vi "TI sbRIO Main (FPGA).vi"() -> ()   [LabVIEW 2019]
uses:
  <userlib>/_NI SPI IP/FPGA/Controllers/Public/Transfer Settings.ctl
  Type Defs/Diagnostic Mode.ctl
  Controls/SPI Channels.ctl
  <vilib>/Platform/TimedLoop/XDataNode/timing_clust.ctl
  <vilib>/Platform/TimedLoop/XDataNode/nitl_modes.ctl
  <vilib>/Platform/TimedLoop/XDataNode/wakeup.ctl
  <vilib>/rvi/FXPMathLib/FxpDiv/subVIs/nifxpmath_Div_SimConfig.ctl
  <vilib>/rvi/FXPMathLib/basic elements/FxpIntAccumulator/subVIs/nifxpmath_IntAccumulator_SimConfig.ctl
  <vilib>/rvi/FXPMathLib/FxpSqrt/subVIs/nifxpmath_Sqrt_SimConfig.ctl
  <vilib>/fxp/LVFixedPointOverflowPolicyTypeDef.ctl
  <userlib>/_NI SPI IP/FPGA/Controllers/Public/Spi Master Inputs.ctl
  <vilib>/rvi/Emulation/niFpgaGetClockAttributes.vi
  <vilib>/rvi/Emulation/niFpgaSctlEmulationGetInTimedLoop.vi
  <vilib>/rvi/Emulation/niFpgaEmulationReportErrorSimple.vi
  <vilib>/rvi/eio/common/nirviEmuTemplateMethod_errors.vi
  Onboard AIs Global.vi
  <vilib>/rvi/Emulation/niFpgaProcessEmulError.vi
  <vilib>/rvi/Emulation/niFpgaCriticalErrorInLSC.vi
  ADC AI Global.vi
  <vilib>/rvi/FXPMathLib/FxpDiv/simVIs/DllFxpDivTemp_sub.vi
  <vilib>/rvi/DataTransferAndStorage/Container/Common/niFpgaContainerExecOnDevCompGetState.vi
  <vilib>/rvi/Emulation/niFpgaEmulationIsFPGAContextNoSignature.vi
  <vilib>/rvi/errors/niFpgaSetErrorForExecOnDevCompSimple.vi
  <vilib>/rvi/eio/common/nirviEmuReportErrorAndStop.vi
  <vilib>/rvi/DataTransferAndStorage/Container/Common/niFpgaContainerGetUniqueNameForEmu.vi
  <vilib>/rvi/FIFO/Fifo_Resource/nirvififoEmulationSetSize.vi
  <vilib>/rvi/FIFO/Fifo_Resource/nirviFifoEmulationQueueMgr.vi
  <instcachedir>/0/nirviFifoEmulationQueueMgr_E5CAEC123FF24DC58D834DCA3CDAA9B5.lvgen/nirviFifoEmulationQueueMgr_E5CAEC123FF24DC58D834DCA3CDAA9B5_000.vi
  <vilib>/rvi/FIFO/Fifo_Resource/nirvififoEmulationDetermineInputValidOut.vi
  <vilib>/rvi/FIFO/Fifo_Resource/nirvififoEmulationCreateLock.vi
  <vilib>/rvi/FIFO/Fifo_Resource/nirvififoEmulationObtainLock.vi
  <vilib>/rvi/FIFO/Fifo_Resource/nirvififoEmulationReleaseLock.vi
  <vilib>/rvi/occurrence/nirviWaitOnOccurrenceBase.vi
  <vilib>/rvi/errors/nirviReportUnexpectedCaseInternalError.vi
  <vilib>/rvi/errors/nirviReportUnexpectedCaseInternalError (U32).vi
  <vilib>/Utility/error.llb/Clear Errors.vi
  <vilib>/rvi/interface/RandomDataEmulation/niFpgaRandomDataHandleErrors.vi
  Diagnostic Global.vi
  Diagnostic Global (U32).vi
  Flow Frequencies Global.vi
  ADC AI Global (Avg).vi
  <vilib>/rvi/Analysis/common/codeGenErrors/XNode/niFpgaXNodeCodeGenErrorHandle.vi
  <vilib>/rvi/FXPMathLib/basic elements/FxpIntAccumulator/simVIs/DllFxpIntAccumulator_sub.vi
  <vilib>/rvi/FXPMathLib/FxpSqrt/simVIs/DllSqrtTemp_sub.vi
  Pump Currents Global.vi
  ADC AI Global (U32).vi
  <vilib>/eio/EIONode/EIONode.xnode
  <vilib>/rvi/FXPMathLib/FxpDiv/XNode/nifxpmath_Div.xnode
  <vilib>/rvi/DataTransferAndStorage/Container/XNode/niFpgaContainer.xnode
  <vilib>/rvi/FIFO/Fifo_Resource/niFpgaFifoEmulationRefIn.vi
  <vilib>/rvi/FXPMathLib/FxpMul/XNode/nifxpmath_Multiplier.xnode
  <vilib>/rvi/FXPMathLib/FxpAdd/XNode/nifxpmath_Add.xnode
  <vilib>/rvi/Analysis/measure/butterworth/XNode/niFpgaButterworthFilter.xnode
  <vilib>/rvi/Analysis/measure/dc-rms/XNode/niFpgaDC-RMS.xnode
  <vilib>/Platform/TimedLoop/XDataNode/XDataNode.xnode
  <vilib>/rvi/FXPMathLib/basic elements/FxpIntAccumulator/XNode/nifxpmath_IntAccumulator.xnode
  <vilib>/rvi/FXPMathLib/FxpSqrt/XNode/nifxpmath_Sqrt.xnode
  <vilib>/rvi/interface/RandomDataEmulation/nirviRandomDataFpgaReadWriteTemplate.vi
  <vilib>/eio/EIOMethodNode/EIOMethodNode.xnode
  <vilib>/rvi/FXPMathLib/sim/FxpSim.dll
  <vilib>/Platform/TimedLoop/XDataNode/XDNodeRunTimeDep.lvlib
  <userlib>/_NI SPI IP/FPGA/Controllers/NI SPI IP FPGA.lvlib
panel:
  out "Pump Cmds":fxp<+/-,28,17>[](array[numeric])
  in  "Pumps Present":bool[](array[boolean])=[FALSE, FALSE, FALSE, FALSE, FALSE, FALSE]
  in  "Pump Cmds (Duty)":u32[](array[numeric])=[0, 0, 0, 0, 0, 0]
  in  "Debug Restarts":bool
  out "Pump No Starts":u32[](array[numeric])
  in  "Initial No Starts":u32[](array[numeric])=[0, 0, 0, 0, 0, 0]
  in  "Pump Start Time":u32
  out "Restarts":i32[](array[numeric])
  out "Cmd Pump Starts":u32[](array[numeric])
  in  "Stop Command":i32
  in  "Initial Cmd Starts":u32[](array[numeric])=[0, 0, 0, 0, 0, 0]
  in  "Ctrl Currents":fxp<+/-,28,17>[](array[numeric])=[0.0, 0.0, 0.0, 0.0, 0.0, 0.0]
  in  "Initial Acutal Starts":u32[](array[numeric])=[0, 0, 0, 0, 0, 0]
  in  "Power Relays":bool[](array[boolean])=[FALSE, FALSE, FALSE, FALSE, FALSE, FALSE]
  out "Actual Pump Starts":u32[](array[numeric])
  out "Timers (ms)":u32[](array[numeric])
  out "Pump On States":bool[](array[boolean])
  in  "Off Current Thresh":fxp<+/-,28,17>
  in  "Min Off Time":u32
  in  "On Current Thresh":fxp<+/-,28,17>
  in  "Min On Time":u32
  in  "Reset Pump Starts":bool
  in  "Pump Starts Enable":bool
  in  "Diag Max Period (ticks)":u32
  in  "Diagnostic Mode":T1=enum."PSA"
  in  "Duty (Ticks)":i32[](array[numeric])=[0, 0, 0, 0, 0, 0]
  out "Elapsed Times OUT":fxp<+,40,40>[](array[numeric])
  out "Data OUT":fxp<+/-,28,17>[](array[numeric])
  in  "Diagnostic Filter":u16=5
  in  "Invert Diagnostic":bool
  in  "Diagnostic Freq Coeff":i32
  in  "Count Off-Time":bool
  in  "Elapsed Times":fxp<+,40,40>[](array[numeric])=[0.0, 0.0, 0.0, 0.0, 0.0, 0.0]
  in  "ADC Init":bool=TRUE
  in  "FFT_Amp?":bool=TRUE
  in  "Max Period (ticks)":u32
  in  "Freq Flow?":bool
  in  "Divide Value":u8=1
  in  "Current Threshold":fxp<+,26,7>=1.0 format="%#_22g"
  in  "Enable Timers":bool[](array[boolean])=[FALSE, FALSE, FALSE, FALSE, FALSE, FALSE]
  in  "PumpCurrentM":fxp<+/-,16,9>=-60.0 format="%#_25g"
  in  "PumpCurrentB":fxp<+/-,16,9>=-60.0 format="%#_25g"
  in  "InvertPWM?":bool
  in  "DIO25":bool
  in  "DIO24":bool
  out "DIO23":bool
  in  "DIO22":bool
  in  "DIO21":bool
  in  "DIO20":bool
  in  "DIO19":bool
  in  "DIO18":bool
  in  "DIO17":bool
  in  "DIO16":bool
  in  "DIO15":bool
  in  "DIO14":bool
  in  "DIO13":bool
  in  "DIO12":bool
  out "ADC Read Data":u64 format="%.0x"
  in  "ADC CS Mode":enum16{"All", "CS0", "CS1"}(ring)
  in  "ADC Trigger":bool=TRUE
  in  "ADC SPI Settings":T2 {"Direction Change Bit" max=64 step=1; "Transfer Length (bits)" min=1 max=64 step=1}
  in  "ADC Data In":u64 format="%.0x"
  in  "ADC Conversion Request":bool
  in  "ADC Manual":bool
  in  "Brushless":bool
  in  "AI Divisor":u32
  in  "AO3":fxp<+/-,20,5>
  in  "AO2":fxp<+/-,20,5>
  in  "Pressure Cmd":fxp<+/-,20,5>
  in  "PS Cmd":fxp<+/-,20,5>
  in  "Loop Timer (uSec)":u32=100
  in  "Timer Resets":bool[](array[boolean])=[FALSE, FALSE, FALSE, FALSE, FALSE, FALSE]
  in  "PWM Period (Ticks)":u32=40000000
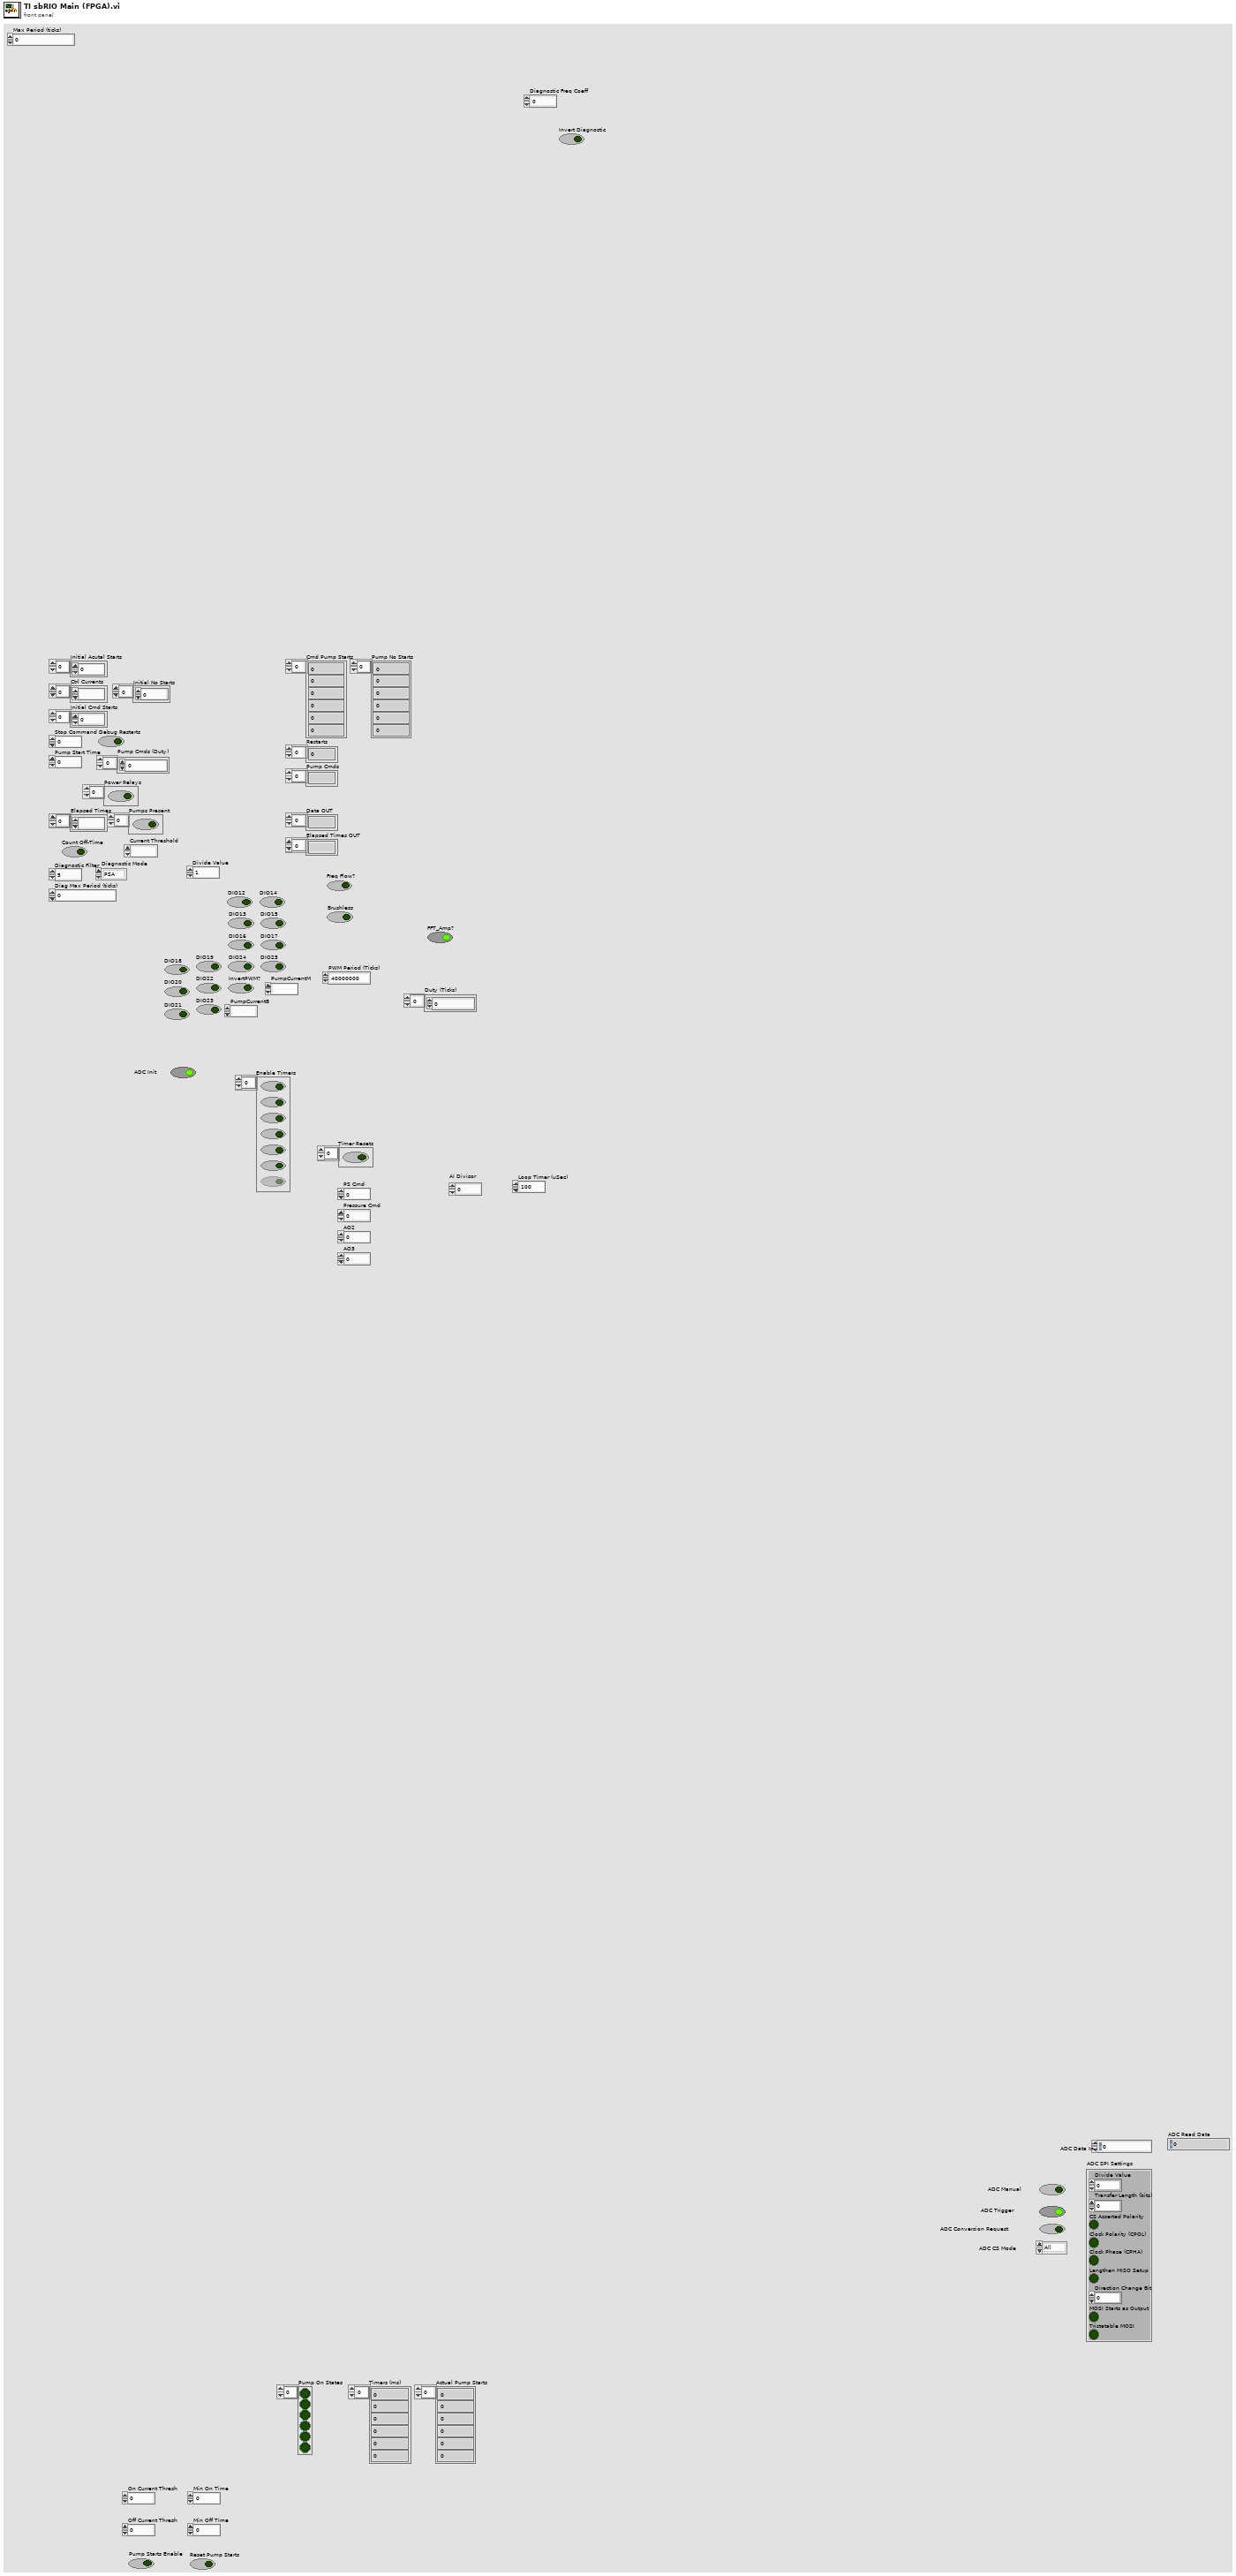
[diagram p1: front panel]
types:
  T1 = typedef "Diagnostic Mode.ctl" = enum16{"None", "PSA", "CMFB"}
  T2 = typedef "NI SPI IP FPGA.lvlib/Transfer Settings.ctl" = cluster{"Divide Value":u8, "Transfer Length (bits)":u8, "CS Asserted Polarity":bool, "Clock Polarity (CPOL)":bool, "Clock Phase (CPHA)":bool, "Lengthen MISO Setup":bool, "Direction Change Bit":u8, "MOSI Starts as Output":bool, "Tristatable MOSI":bool}
  T3 = typedef "SPI Channels.ctl" = cluster{"CS":refnum<k21>, "CLK":refnum<k21>, "MOSI":refnum<k21>, "MISO":refnum<k21>}
  T4 = typedef "XDNodeRunTimeDep.lvlib/timing_clust.ctl" = cluster{"Expected End [f-1]":u64, "Actual End [f-1]":u64, "Finished Late? [f-1]":bool, "Expected End [i-1]":u64, "Actual End [i-1]":u64, "Finished Late? [i-1]":bool, "Expected Start [i]":u64, "Actual Start [i]":u64, "Expected Start [f]":u64, "Actual Start [f]":u64, "Source Name":string, "Structure Name":string, "Period":i64, "Deadline":i64, "Offset":i64, "Start":i64, "Priority":i32, "Timeout":i32, "Mode":T5, "Wakeup Reason":T6, "Error":errorcluster, "Source Type":string, "Secondary Source Type":string, "Global End Time":u64, "Global Start Time":u64, "Frame Duration":u64, "Iteration Duration":u64, "Assigned CPU":i32, "I/O Scan Engine Mode":u32}
  T5 = typedef "XDNodeRunTimeDep.lvlib/nitl_modes.ctl" = enum32{"No Change", "Process missed periods, maintain original phase", "Discard missed periods, maintain original phase", "Process missed periods, ignore original phase", "Discard missed periods, ignore original phase"}
  T6 = typedef "XDNodeRunTimeDep.lvlib/wakeup.ctl" = enum32{"Normal", "Aborted", "Asynchronous wakeup", "Timing source error", "Timed loop error", "Timeout"}
  T7 = typedef "NI SPI IP FPGA.lvlib/Spi Master Inputs.ctl" = cluster{"MISO":bool}
  T8 = typedef "NI SPI IP FPGA.lvlib/Spi Master Outputs.ctl" = cluster{"Chip Select":bool, "Clock":bool, "MOSI":bool, "MOSI OE":bool}
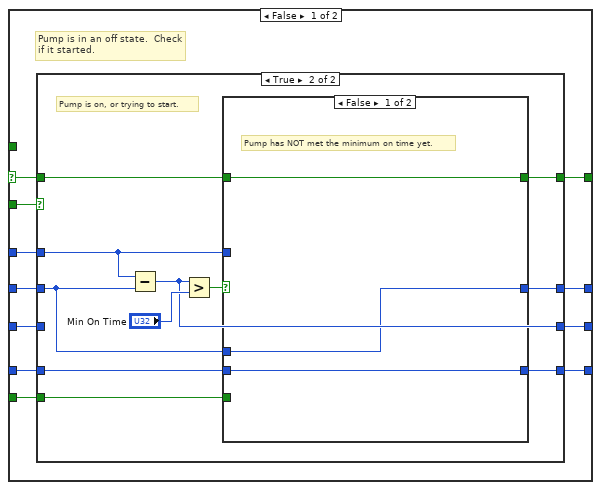
[diagram p6: hidden frame]
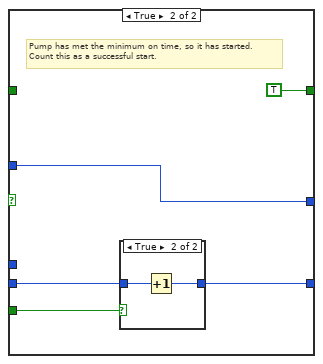
[diagram p8: hidden frame]
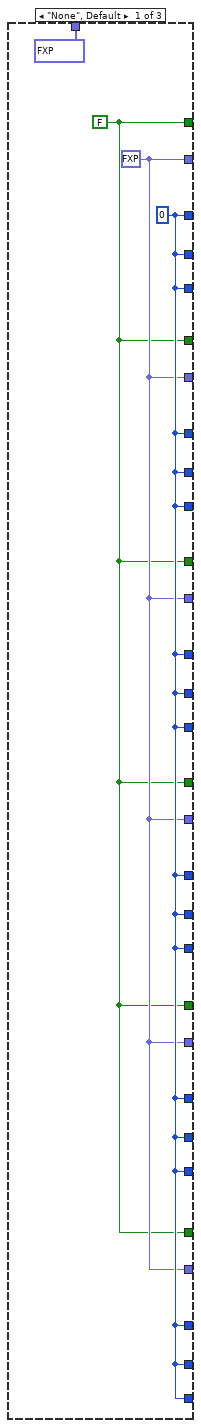
[diagram p12: hidden frame]
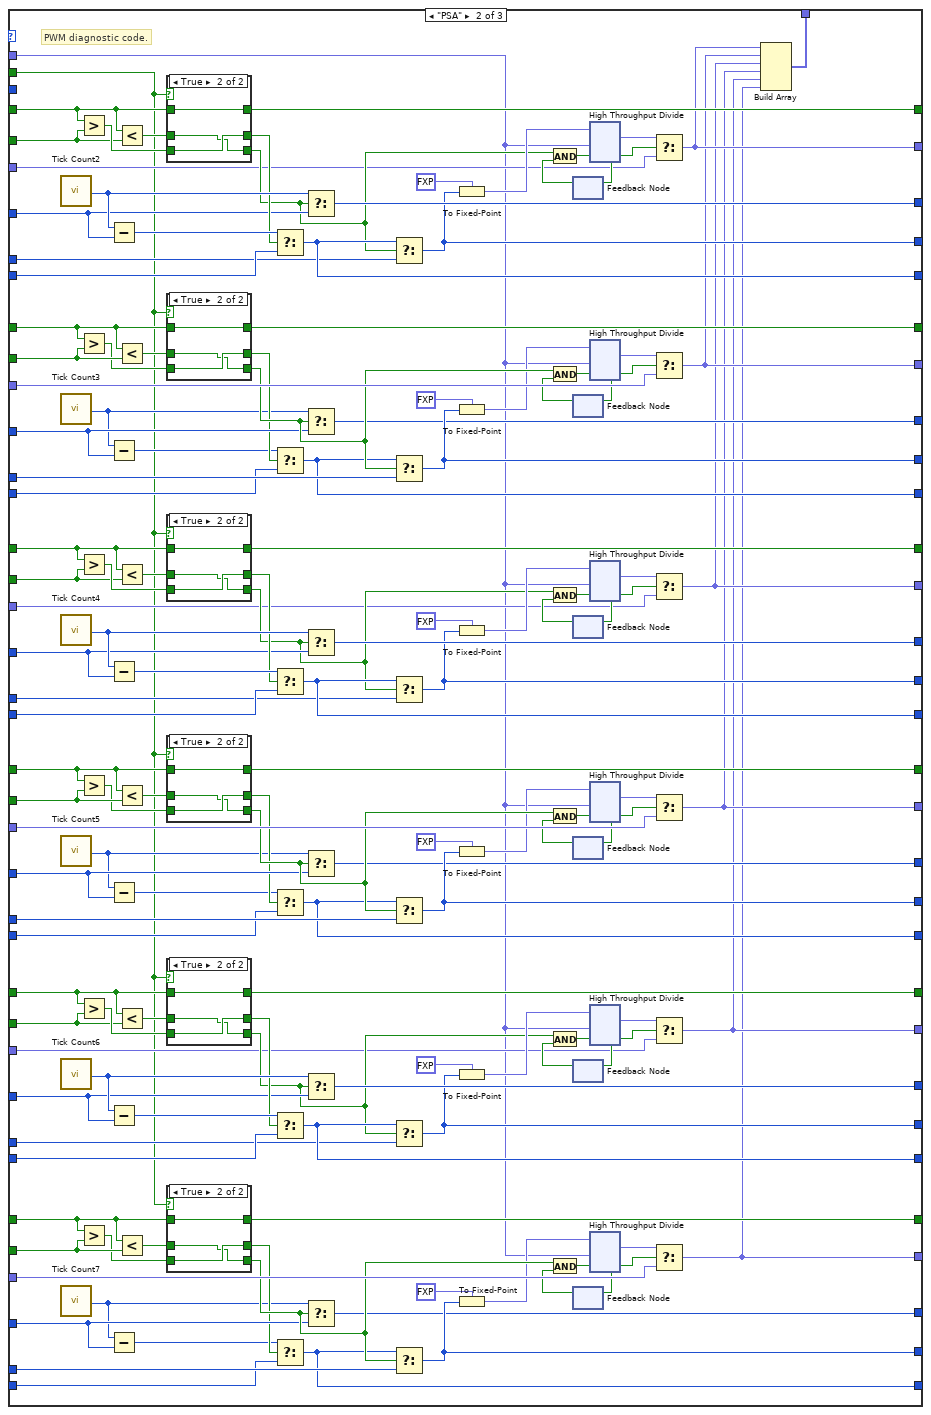
[diagram p13: hidden frame]
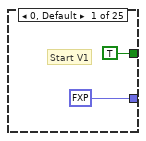
[diagram p20: hidden frame]
diagram:
  w4 = bool[] [FALSE, FALSE, FALSE, FALSE, FALSE, FALSE]  # Pump Triggered
  w10 = bool[] [FALSE, FALSE, FALSE, FALSE, FALSE, FALSE]  # Pump On States
  w41 = refnum<k21> "RMC/DIO60"  # CONVST
  w42 = refnum<k21> "RMC/DIO59"  # CDI
  w43 = refnum<k21> "RMC/DIO58"  # CS1
  w47 = u8 31 ("Sample Divisor")
  # "Pump Start Monitor (for finding restarts)."
  # "DMA for crash files."
  # "Main source of data for RT."
  # "Pump Phase Current and Elapsed Times."
  # "PWM Outputs for Controller Command."
  # "Signal Averaging."
  # "FFT for Pump Speed."
  # "Pump Controller Diagnostics."
  # "Turbine Flow Meters."
  # "Control Signals"
  # "4x ADC\n\nAI16\tPump Current 1\nAI17\tPump Current 2\nAI18\tPump Current 3\nAI19\tPump Current 4\nAI20\tPump Current 5\nAI21\tPump Current 6\nAI22\tController Current 1\nAI23\tController Current 2\nAI24\tController Current 3\nAI25\tController Current 4\nAI26\tController Current 5\nAI27\tController Current 6\nAI28\tTemp 1\nAI29\tTemp 2\nAI30\tPump Pressure 1\nAI31\tPump Pressure 2\nAI32\tPump Pressure 3\nAI33\tPump Pressure 4\nAI34\tPump Pressure 5\nAI35\tPump Pressure 6\nAI36\tPump Flow 1\nAI37\tPump Flow 2\nAI38\tPump Flow 3\nAI39\tPump Flow 4\nAI40\tPump Flow 5\nAI41\tPump Flow 6\nAI42\tSpare\nAI43\tSpare\nAI44\tSpare\nAI45\tSpare\nAI46\tSpare\nAI47\tSpare"
  # "Onboard\n\nAI0/8\tVoltage 1\nAI1/9\tVoltage 2\nAI2/10\tVoltage 3\nAI3/11\tVoltage 4\nAI4/12\tVoltage 5\nAI5/13\tVoltage 6\nAI6\tSpare\nAI14\tSpare\nAI7\tSpare\nAI15\tPower Supply Sense"
  # "This code was created to use\nwith an 8ch analog input to SPI\nchip (ADS8332IPW)."
  # "Explanation for Rounding http://www.eetimes.com/document.asp?doc_id=1274485&page_number=1"
  # "Explanation of Saturation vs. wrapping:   http://www.mathworks.com/help/fixedpoint/ug/saturation-and-wrapping.html\n If scale is 0 to 8 and value is -2               Saturation: 0    Wrapping:  6"
  n1 = node-c288() -> (w32:T4)  [unwired: 1 in]
  n2 = node-c288() -> (w30:T4)  [unwired: 1 in]
  n3 = Unbundle By Name(T3 {"CS"="RMC/DIO57", "CLK"="RMC/DIO54", "MOSI"="RMC/DIO56", "MISO"="RMC/DIO55"} ("SPI Channels")) -> ("CS"=w34:refnum<k21>, "CLK"=w35:refnum<k21>, "MOSI"=w36:refnum<k21>, "MISO"=w37:refnum<k21>)
  n4 = call "Tick Count8"() -> ("Tick Count(mSec)"=w7:u32)
  n5 = timed-loop {
    timing: w32 -> [_]
    timing-out: [_] -> w31
    stop <- FALSE stop-if-true
    n6 = Index Array(array="Power Relays") -> (element #1=w57:bool, element #2=w56:bool, element #3=w55:bool, element #4=w54:bool, element #5=w53:bool, element #6=w52:bool)  [unwired: 6 in]
    n7 = xnode "FPGA I/O Node"("RMC/DIO6"=w57, "RMC/DIO7"=w56, "RMC/DIO8"=w55, "RMC/DIO9"=w54, "RMC/DIO10"=w53, "RMC/DIO11"=w52, "RMC/DIO12"="DIO12", "RMC/DIO13"="DIO13", "RMC/DIO14"="DIO14", "RMC/DIO15"="DIO15", "RMC/DIO16"="DIO16", "RMC/DIO17"="DIO17", "RMC/DIO18"="DIO18", "RMC/DIO19"="DIO19", "RMC/DIO20"="DIO20", "RMC/DIO21"="DIO21", "RMC/DIO22"="DIO22", "RMC/DIO24"="DIO24", "RMC/DIO25"="DIO25") -> ("RMC/DIO23"=→"DIO23":bool)  [unwired: 21 in, 21 out]
  }
  n8 = timed-loop {
    timing: w30 -> [_]
    timing-out: [_] -> w29
    shift-right: [w200] -> _
    shift-left: u32 0 ("f") -> [w199]
    shift-right: [w82] -> _
    shift-left: fxp<+/-,28,17> 0.0 ("AI0") -> [w194]
    shift-right: [w169] -> _
    shift-left: u32 0 ("f") -> [w170]
    shift-right: [w81] -> _
    shift-left: fxp<+/-,28,17> 0.0 ("AI0") -> [w175]
    shift-right: [w160] -> _
    shift-left: u32 0 ("f") -> [w159]
    shift-right: [w80] -> _
    shift-left: fxp<+/-,28,17> 0.0 ("AI0") -> [w154]
    shift-right: [w129] -> _
    shift-left: u32 0 ("f") -> [w130]
    shift-right: [w79] -> _
    shift-left: fxp<+/-,28,17> 0.0 ("AI0") -> [w135]
    shift-right: [w120] -> _
    shift-left: u32 0 ("f") -> [w119]
    shift-right: [w78] -> _
    shift-left: fxp<+/-,28,17> 0.0 ("AI0") -> [w114]
    shift-right: [w89] -> _
    shift-left: u32 0 ("f") -> [w90]
    shift-right: [w77] -> _
    shift-left: fxp<+/-,28,17> 0.0 ("AI0") -> [w95]
    stop <- FALSE stop-if-true
    w84 = fxp<+,32,32> 40000000.0 ("x")
    n9 = xnode "FPGA I/O Node"() -> ("RMC/DIO32"=w204:bool)  [unwired: 1 in, 1 out]
    n10 = xnode "FPGA I/O Node"() -> ("RMC/DIO33"=w165:bool)  [unwired: 1 in, 1 out]
    n11 = xnode "FPGA I/O Node"() -> ("RMC/DIO34"=w164:bool)  [unwired: 1 in, 1 out]
    n12 = xnode "FPGA I/O Node"() -> ("RMC/DIO35"=w125:bool)  [unwired: 1 in, 1 out]
    n13 = xnode "FPGA I/O Node"() -> ("RMC/DIO36"=w124:bool)  [unwired: 1 in, 1 out]
    n14 = xnode "FPGA I/O Node"() -> ("RMC/DIO37"=w85:bool)  [unwired: 1 in, 1 out]
    n15 = feedback-in #1(w204) -> ()
    n16 = feedback #1() -> (w203:bool)  [unwired: 1 in]
    n17 = feedback #2() -> (w166:bool)  [unwired: 1 in]
    n18 = feedback-in #2(w165) -> ()
    n19 = feedback #3() -> (w163:bool)  [unwired: 1 in]
    n20 = feedback-in #3(w164) -> ()
    n21 = feedback #4() -> (w126:bool)  [unwired: 1 in]
    n22 = feedback-in #4(w125) -> ()
    n23 = feedback #5() -> (w123:bool)  [unwired: 1 in]
    n24 = feedback-in #5(w124) -> ()
    n25 = feedback #6() -> (w86:bool)  [unwired: 1 in]
    n26 = feedback-in #6(w85) -> ()
    n27 = Increment(x=w199) -> (x+1=w198:u32)
    n28 = Increment(x=w170) -> (x+1=w171:u32)
    n29 = Increment(x=w159) -> (x+1=w158:u32)
    n30 = Increment(x=w130) -> (x+1=w131:u32)
    n31 = Increment(x=w119) -> (x+1=w118:u32)
    n32 = Increment(x=w90) -> (x+1=w91:u32)
    n33 = Greater?(x=w204, y=w203) -> (0:w185:bool)
    n34 = Greater?(x=w165, y=w166) -> (0:w184:bool)
    n35 = Greater?(x=w164, y=w163) -> (0:w145:bool)
    n36 = Greater?(x=w125, y=w126) -> (0:w144:bool)
    n37 = Greater?(x=w124, y=w123) -> (0:w105:bool)
    n38 = Greater?(x=w85, y=w86) -> (0:w104:bool)
    n39 = Greater?(x=w198, y="Max Period (ticks)") -> (0:w202:bool)
    n40 = Greater?(x=w171, y="Max Period (ticks)") -> (0:w167:bool)
    n41 = Greater?(x=w158, y="Max Period (ticks)") -> (0:w162:bool)
    n42 = Greater?(x=w131, y="Max Period (ticks)") -> (0:w127:bool)
    n43 = Greater?(x=w118, y="Max Period (ticks)") -> (0:w122:bool)
    n44 = Greater?(x=w91, y="Max Period (ticks)") -> (0:w87:bool)
    n45 = To Fixed-Point(number=w198) -> (fixed-point=w197:fxp<+,32,32>)  [unwired: 1 in]
    n46 = To Fixed-Point(number=w171) -> (fixed-point=w172:fxp<+,32,32>)  [unwired: 1 in]
    n47 = To Fixed-Point(number=w158) -> (fixed-point=w157:fxp<+,32,32>)  [unwired: 1 in]
    n48 = To Fixed-Point(number=w131) -> (fixed-point=w132:fxp<+,32,32>)  [unwired: 1 in]
    n49 = To Fixed-Point(number=w118) -> (fixed-point=w117:fxp<+,32,32>)  [unwired: 1 in]
    n50 = To Fixed-Point(number=w91) -> (fixed-point=w92:fxp<+,32,32>)  [unwired: 1 in]
    n51 = feedback #7() -> (w186:bool)  [unwired: 1 in]
    n52 = And(x=w185, y=w186) -> (x .and. y?=w187:bool)
    n53 = feedback #8() -> (w183:bool)  [unwired: 1 in]
    n54 = And(x=w184, y=w183) -> (x .and. y?=w182:bool)
    n55 = feedback #9() -> (w146:bool)  [unwired: 1 in]
    n56 = And(x=w145, y=w146) -> (x .and. y?=w147:bool)
    n57 = feedback #10() -> (w143:bool)  [unwired: 1 in]
    n58 = And(x=w144, y=w143) -> (x .and. y?=w142:bool)
    n59 = feedback #11() -> (w106:bool)  [unwired: 1 in]
    n60 = And(x=w105, y=w106) -> (x .and. y?=w107:bool)
    n61 = feedback #12() -> (w103:bool)  [unwired: 1 in]
    n62 = And(x=w104, y=w103) -> (x .and. y?=w102:bool)
    n63 = xnode "High Throughput Divide"("x"=w84, "y"=w197, "input valid"=w187) -> ("x/y"=w193:fxp<+,28,17>, "output valid"=w189:bool, "ready for input"=w188:bool)  [unwired: 1 in]
    n64 = feedback-in #7(w188) -> ()
    n65 = xnode "High Throughput Divide"("x"=w84, "y"=w172, "input valid"=w182) -> ("x/y"=w176:fxp<+,28,17>, "output valid"=w180:bool, "ready for input"=w181:bool)  [unwired: 1 in]
    n66 = feedback-in #8(w181) -> ()
    n67 = xnode "High Throughput Divide"("x"=w84, "y"=w157, "input valid"=w147) -> ("x/y"=w153:fxp<+,28,17>, "output valid"=w149:bool, "ready for input"=w148:bool)  [unwired: 1 in]
    n68 = feedback-in #9(w148) -> ()
    n69 = xnode "High Throughput Divide"("x"=w84, "y"=w132, "input valid"=w142) -> ("x/y"=w136:fxp<+,28,17>, "output valid"=w140:bool, "ready for input"=w141:bool)  [unwired: 1 in]
    n70 = feedback-in #10(w141) -> ()
    n71 = xnode "High Throughput Divide"("x"=w84, "y"=w117, "input valid"=w107) -> ("x/y"=w113:fxp<+,28,17>, "output valid"=w109:bool, "ready for input"=w108:bool)  [unwired: 1 in]
    n72 = feedback-in #11(w108) -> ()
    n73 = xnode "High Throughput Divide"("x"=w84, "y"=w92, "input valid"=w102) -> ("x/y"=w96:fxp<+,28,17>, "output valid"=w100:bool, "ready for input"=w101:bool)  [unwired: 1 in]
    n74 = feedback-in #12(w101) -> ()
    n75 = Select(t=u32 0 ("f"), s=w189, f=w198) -> (s? t:f=w200:u32)
    n76 = Select(t=u32 0 ("f"), s=w180, f=w171) -> (s? t:f=w169:u32)
    n77 = Select(t=u32 0 ("f"), s=w149, f=w158) -> (s? t:f=w160:u32)
    n78 = Select(t=u32 0 ("f"), s=w140, f=w131) -> (s? t:f=w129:u32)
    n79 = Select(t=u32 0 ("f"), s=w109, f=w118) -> (s? t:f=w120:u32)
    n80 = Select(t=u32 0 ("f"), s=w100, f=w91) -> (s? t:f=w89:u32)
    n81 = To Fixed-Point(fixed-point type=fxp<+/-,28,17> 0.0 ("AI0"), number=w193) -> (fixed-point=w191:fxp<+/-,28,17>)
    n82 = To Fixed-Point(fixed-point type=fxp<+/-,28,17> 0.0 ("AI0"), number=w176) -> (fixed-point=w178:fxp<+/-,28,17>)
    n83 = To Fixed-Point(fixed-point type=fxp<+/-,28,17> 0.0 ("AI0"), number=w153) -> (fixed-point=w151:fxp<+/-,28,17>)
    n84 = To Fixed-Point(fixed-point type=fxp<+/-,28,17> 0.0 ("AI0"), number=w136) -> (fixed-point=w138:fxp<+/-,28,17>)
    n85 = To Fixed-Point(fixed-point type=fxp<+/-,28,17> 0.0 ("AI0"), number=w113) -> (fixed-point=w111:fxp<+/-,28,17>)
    n86 = To Fixed-Point(fixed-point type=fxp<+/-,28,17> 0.0 ("AI0"), number=w96) -> (fixed-point=w98:fxp<+/-,28,17>)
    n87 = Or(x=w202, y=w189) -> (x .or. y?=w195:bool)
    n88 = Or(x=w167, y=w180) -> (x .or. y?=w174:bool)
    n89 = Or(x=w162, y=w149) -> (x .or. y?=w155:bool)
    n90 = Or(x=w127, y=w140) -> (x .or. y?=w134:bool)
    n91 = Or(x=w122, y=w109) -> (x .or. y?=w115:bool)
    n92 = Or(x=w87, y=w100) -> (x .or. y?=w94:bool)
    n93 = Select(t=fxp<+/-,28,17> 0.0 ("AI0"), s=w202, f=w191) -> (s? t:f=w196:fxp<+/-,28,17>)
    n94 = Select(t=fxp<+/-,28,17> 0.0 ("AI0"), s=w167, f=w178) -> (s? t:f=w173:fxp<+/-,28,17>)
    n95 = Select(t=fxp<+/-,28,17> 0.0 ("AI0"), s=w162, f=w151) -> (s? t:f=w156:fxp<+/-,28,17>)
    n96 = Select(t=fxp<+/-,28,17> 0.0 ("AI0"), s=w127, f=w138) -> (s? t:f=w133:fxp<+/-,28,17>)
    n97 = Select(t=fxp<+/-,28,17> 0.0 ("AI0"), s=w122, f=w111) -> (s? t:f=w116:fxp<+/-,28,17>)
    n98 = Select(t=fxp<+/-,28,17> 0.0 ("AI0"), s=w87, f=w98) -> (s? t:f=w93:fxp<+/-,28,17>)
    n99 = Select(t=w196, s=w195, f=w194) -> (s? t:f=w82:fxp<+/-,28,17>)
    n100 = Select(t=w173, s=w174, f=w175) -> (s? t:f=w81:fxp<+/-,28,17>)
    n101 = Select(t=w156, s=w155, f=w154) -> (s? t:f=w80:fxp<+/-,28,17>)
    n102 = Select(t=w133, s=w134, f=w135) -> (s? t:f=w79:fxp<+/-,28,17>)
    n103 = Select(t=w116, s=w115, f=w114) -> (s? t:f=w78:fxp<+/-,28,17>)
    n104 = Select(t=w93, s=w94, f=w95) -> (s? t:f=w77:fxp<+/-,28,17>)
    n105 = Build Array(w82, w81, w80, w79, w78, w77) -> (w76:fxp<+/-,28,17>[])
    n106 = global write "Flow Frequencies Global.vi" "Flow Frequencies"(w76) -> ()
  }
  n107 = local read "Duty (Ticks)"() -> (w5:i32[])
  n108 = while {
    shift-right: [w383] -> _
    shift-left: "Elapsed Times" -> [w394]
    shift-right: [w384] -> _
    shift-left: u32[] [0, 0, 0, 0, 0, 0] -> [w385]
    stop <- FALSE stop-if-true
    # "Pump Current\nAI16-21"
    # "from:S 64 44\nto: U 40 40"
    n109 = global read "ADC AI Global.vi" "AI16-47"() -> (w387:fxp<+/-,28,17>[])
    n110 = feedback #13() -> (w392:bool[])  [unwired: 1 in]
    n111 = feedback-in #13("Timer Resets") -> ()
    n112 = Array Subset(array=w387, index=0, length=6) -> (w389:fxp<+/-,28,17>[])
    n113 = Greater?(x="Timer Resets", y=w392) -> (0:w395:bool[])
    n114 = for {
      tunnel: w389 -> [w429] mode=indexing
      tunnel: w395 -> [w431] mode=indexing
      tunnel: [w401] -> w386 mode=indexing
      tunnel: w394 -> [w426] mode=indexing
      tunnel: [w425] -> w383 mode=indexing
      tunnel: "Enable Timers" -> [w420] mode=indexing
      tunnel: w385 -> [w408] mode=indexing
      tunnel: [w403] -> w384 mode=indexing
      tunnel: "Count Off-Time" -> [w399]
      i -> [w430]
      w424 = fxp<+/-,26,7> 0.0 ("out")
      # "Formerly looking for DC signal based on period detection\nNow looking for staying in the 0A range"
      # "Calibration issue should only\nbe if reading is negative at 0A"
      # "30ms calculated as longest waveform period"
      # "RMS vi only outputs positive values, so put back to negative if that's the way it went in.  This fixes a calibration issue."
      # "D2A factor"
      # "Rough scale and offset for\nspeed and RMS measurements."
      n115 = xnode "High Throughput Divide"("x"=w429, "y"=fxp<+,14,14> 13107.0 ("Current Scale")) -> ("x/y"=w423:fxp<+/-,28,17>)
      n116 = xnode ("High Throughput Multiply")("x"=w423, "y"="PumpCurrentM") -> ("x*y"=w422:fxp<+/-,29,10>)
      n117 = xnode ("High Throughput Add")("x"=w422, "y"="PumpCurrentB") -> ("x+y"=w411:fxp<+/-,30,11>)
      n118 = Less?(x=w411, y=fxp<+/-,30,11> 0.25) -> (x < y?=w409:bool)
      n119 = xnode "Butterworth Filter"("input data"=w411) -> ("output data"=w413:fxp<+/-,20,15>)  [unwired: 2 in, 1 out]
      n120 = case shown="True" w409 {
        tunnel: w408 -> [_ w434]
        tunnel: [u32 0 w433] -> w403
        frame False {
        }
        frame True {
          n121 = Increment(x=w434) -> (x+1=w433:u32)
        }
      }
      n122 = To Fixed-Point(fixed-point type=w424, number=w411) -> (fixed-point=w416:fxp<+/-,26,7>)
      n123 = To Fixed-Point(fixed-point type=w424, number=w413) -> (fixed-point=w414:fxp<+/-,26,7>)
      n124 = case shown="False" "Brushless" {
        tunnel: [w435 w436] -> w415
        tunnel: w416 -> [_ w436]
        tunnel: w414 -> [w435 _]
        frame False {
        }
        frame True {
        }
      }
      n125 = Greater?(x=w403, y=u32 300) -> (0:w404:bool)
      n126 = Less Than 0?(x=w415) -> (x < 0?=w407:bool)
      n127 = case shown="0, Default" w430 {
        tunnel: [w490 w600 w710 w820 w930 w1040] -> w417
        tunnel: w415 -> [w489 w599 w709 w819 w929 w1039]
        frame 0, Default {
          n128 = xnode ("DC and RMS Measurements 5")("input data"=w489) -> ("RMS"=w490:fxp<+,26,7>)  [unwired: 1 in, 1 out]
        }
        frame 1 {
          n129 = xnode ("DC and RMS Measurements")("input data"=w599) -> ("RMS"=w600:fxp<+,26,7>)  [unwired: 1 in, 1 out]
        }
        frame 2 {
          n130 = xnode ("DC and RMS Measurements 2")("input data"=w709) -> ("RMS"=w710:fxp<+,26,7>)  [unwired: 1 in, 1 out]
        }
        frame 3 {
          n131 = xnode ("DC and RMS Measurements 3")("input data"=w819) -> ("RMS"=w820:fxp<+,26,7>)  [unwired: 1 in, 1 out]
        }
        frame 4 {
          n132 = xnode ("DC and RMS Measurements 4")("input data"=w929) -> ("RMS"=w930:fxp<+,26,7>)  [unwired: 1 in, 1 out]
        }
        frame 5 {
          n133 = xnode ("DC and RMS Measurements 6")("input data"=w1039) -> ("RMS"=w1040:fxp<+,26,7>)  [unwired: 1 in, 1 out]
        }
      }
      n134 = And(x=w407, y=w404) -> (x .and. y?=w406:bool)
      n135 = To Fixed-Point(fixed-point type=fxp<+/-,28,17> 0.0 ("out"), number=w417) -> (fixed-point=w418:fxp<+/-,28,17>)
      n136 = case shown="True" w406 {
        tunnel: w418 -> [w437 w439]
        tunnel: [w437 w438] -> w401
        frame False {
        }
        frame True {
          n137 = Negate(x=w439) -> (-x=w438:fxp<+/-,29,18>)
        }
      }
      n138 = Greater?(x=w401, y="Current Threshold") -> (0:w400:bool)
      n139 = Or(x=w400, y=w399) -> (x .or. y?=w398:bool)
      n140 = case shown="True" w431 {
        tunnel: w398 -> [w470 _]
        tunnel: w426 -> [w469 _]
        tunnel: [w468 fxp<+,40,40> 0.0 ("AI0")] -> w425
        tunnel: w420 -> [w467 _]
        frame False {
          n141 = case shown="True" w467 {
            tunnel: w470 -> [_ w474]
            tunnel: w469 -> [w471 w473]
            tunnel: [w471 w472] -> w468
            frame False {
            }
            frame True {
              n142 = case shown="True" w474 {
                tunnel: [w475 w476] -> w472
                tunnel: w473 -> [w475 w478]
                frame False {
                }
                frame True {
                  # "Was: Sat/Trunc       Now:  Wrap/Trunc"
                  # "Greater than 1 amp, so pump is \"on\"."
                  n143 = xnode ("High Throughput Add")("x"=w478, "y"=fxp<+,1,1> 1.0) -> ("x+y"=w476:fxp<+,40,40>)
                }
              }
            }
          }
        }
        frame True {
        }
      }
    }
    n144 = call "Loop Timer"("Count(uSec)"="Loop Timer (uSec)") -> ()  [unwired: 1 out]
    n145 = global write "Pump Currents Global.vi" "Pump Currents"(w386) -> ()
    n146 = local write "Elapsed Times"(w383) -> ()
  }
  n147 = while {
    stop <- FALSE stop-if-true
    n148 = Index Array(array="Duty (Ticks)") -> (element #1=w1154:i32, element #2=w1153:i32, element #3=w1152:i32, element #4=w1151:i32, element #5=w1150:i32, element #6=w1149:i32)  [unwired: 6 in]
    n149 = call "Pulse Width Modulation (FPGA).vi"("PWM Period (Ticks)"="PWM Period (Ticks)", "PWM Duty Cycle (Ticks)"=w1154) -> ("PWM DO"=w1168:bool)  [unwired: 14 in, 3 out]
    n150 = call "Pulse Width Modulation (FPGA).vi"("PWM Period (Ticks)"="PWM Period (Ticks)", "PWM Duty Cycle (Ticks)"=w1153) -> ("PWM DO"=w1167:bool)  [unwired: 14 in, 3 out]
    n151 = call "Pulse Width Modulation (FPGA).vi"("PWM Period (Ticks)"="PWM Period (Ticks)", "PWM Duty Cycle (Ticks)"=w1152) -> ("PWM DO"=w1166:bool)  [unwired: 14 in, 3 out]
    n152 = call "Pulse Width Modulation (FPGA).vi"("PWM Period (Ticks)"="PWM Period (Ticks)", "PWM Duty Cycle (Ticks)"=w1151) -> ("PWM DO"=w1165:bool)  [unwired: 14 in, 3 out]
    n153 = call "Pulse Width Modulation (FPGA).vi"("PWM Period (Ticks)"="PWM Period (Ticks)", "PWM Duty Cycle (Ticks)"=w1150) -> ("PWM DO"=w1164:bool)  [unwired: 14 in, 3 out]
    n154 = call "Pulse Width Modulation (FPGA).vi"("PWM Period (Ticks)"="PWM Period (Ticks)", "PWM Duty Cycle (Ticks)"=w1149) -> ("PWM DO"=w1163:bool)  [unwired: 14 in, 3 out]
    n155 = Exclusive Or(1:"InvertPWM?", 2:w1168) -> (0:w1161:bool)
    n156 = Exclusive Or(1:"InvertPWM?", 2:w1167) -> (0:w1160:bool)
    n157 = Exclusive Or(1:"InvertPWM?", 2:w1166) -> (0:w1159:bool)
    n158 = Exclusive Or(1:"InvertPWM?", 2:w1165) -> (0:w1158:bool)
    n159 = Exclusive Or(1:"InvertPWM?", 2:w1164) -> (0:w1157:bool)
    n160 = Exclusive Or(1:"InvertPWM?", 2:w1163) -> (0:w1156:bool)
    n161 = xnode "FPGA I/O Node"("RMC/DIO0"=w1161, "RMC/DIO1"=w1160, "RMC/DIO2"=w1159, "RMC/DIO3"=w1158, "RMC/DIO4"=w1157, "RMC/DIO5"=w1156) -> ()  [unwired: 7 in, 7 out]
  }
  n162 = node-c288() -> (w45:T4)  [unwired: 1 in]
  n163 = node-c288() -> (w51:T4)  [unwired: 1 in]
  n164 = node-c288() -> (w12:T4)  [unwired: 1 in]
  n165 = Initialize Array(w7, 6 ("dimension size")) -> (w3:u32[])
  n166 = Decrement(x=w47) -> (x-1=w48:u8)
  n167 = timed-loop "4x ADC SPI Loop" {
    shift-right: [w1195] -> _
    shift-left: fxp<+/-,28,17>[] [0.0, 0.0, 0.0, 0.0, 0.0, 0.0, 0.0, 0.0, 0.0, 0.0, 0.0, 0.0, 0.0, 0.0, 0.0, 0.0, 0.0, 0.0, 0.0, 0.0, 0.0, 0.0, 0.0, 0.0, 0.0, 0.0, 0.0, 0.0, 0.0, 0.0, 0.0, 0.0] -> [w1196]
    tunnel: w34 -> [w1194]
    tunnel: w35 -> [w1193]
    tunnel: w36 -> [w1192]
    tunnel: w37 -> [w1191]
    tunnel: w43 -> [w1190]
    tunnel: w41 -> [w1189]
    tunnel: w42 -> [w1188]
    timing: w45 -> [_]
    timing-out: [_] -> w44
    shift-right: [w1177] -> _
    shift-left: u8 2 ("lo(x)") -> [w1178]
    shift-right: [w1174] -> _
    shift-left: u8 0 ("lo(x)") -> [w1175]
    shift-right: [w1171] -> _
    shift-left: u32[] [0, 0, 0, 0, 0, 0, 0, 0, 0, 0, 0, 0, 0, 0, 0, 0, 0, 0, 0, 0, 0, 0, 0, 0, 0, 0, 0, 0, 0, 0, 0, 0] -> [w1172]
    stop <- FALSE stop-if-true
    n168 = flat-sequence {
      tunnel: [w1209] -> w1187
      tunnel: w1196 -> [w1209]
      tunnel: w1194 -> [w1208]
      tunnel: w1193 -> [w1207]
      tunnel: w1192 -> [w1206]
      tunnel: w1191 -> [w1205]
      tunnel: [w1208] -> w1186
      tunnel: [w1207] -> w1185
      tunnel: [w1206] -> w1184
      tunnel: [w1205] -> w1183
      tunnel: w1190 -> [w1204]
      tunnel: w1189 -> [w1203]
      tunnel: w1188 -> [w1202]
      tunnel: [w1204] -> w1182
      tunnel: [w1202] -> w1181
      tunnel: [w1203] -> w1180
      tunnel: [w1201] -> w1179
      tunnel: w1178 -> [w1201]
      tunnel: [w1200] -> w1176
      tunnel: w1175 -> [w1200]
      tunnel: [w1198] -> w1173
      tunnel: w1172 -> [w1198]
      tunnel: w1187 -> [w1254]
      tunnel: [w1253] -> w1195
      tunnel: w1186 -> [w1249]
      tunnel: w1185 -> [w1252]
      tunnel: w1184 -> [w1251]
      tunnel: w1183 -> [w1250]
      tunnel: w1182 -> [w1248]
      tunnel: w1181 -> [_]
      tunnel: w1180 -> [w1234]
      tunnel: w1179 -> [w1235]
      tunnel: [w1229] -> w1177
      tunnel: w1176 -> [w1228]
      tunnel: [w1227] -> w1174
      tunnel: w1173 -> [w1226]
      tunnel: [w1225] -> w1171
      frame #0 {
        # "Message Type Index"
        n169 = case shown="True" "ADC Init" {
          tunnel: w1208 -> [_ w1224]
          tunnel: w1207 -> [_ w1223]
          tunnel: w1206 -> [_ w1222]
          tunnel: w1205 -> [_ w1221]
          tunnel: w1204 -> [_ w1220]
          tunnel: w1203 -> [_ w1219]
          tunnel: w1202 -> [_ w1218]
          frame False {
          }
          frame True {
            w1211 = TRUE ("I/O Item")
            w1216 = TRUE ("Enable")
            n170 = xnode "FPGA I/O Method Node"("FPGA I/O In"=w1219, "Enable"=w1216) -> ("FPGA I/O Out"=w1212:refnum<k21>)
            n171 = xnode "FPGA I/O Method Node"("FPGA I/O In"=w1218, "Enable"=FALSE) -> ()  [unwired: 1 out]
            n172 = xnode "FPGA I/O Method Node"("FPGA I/O In"=w1220, "Enable"=w1216) -> ("FPGA I/O Out"=w1215:refnum<k21>)
            n173 = xnode "FPGA I/O Method Node"("FPGA I/O In"=w1224, "Enable"=w1216) -> ("FPGA I/O Out"=w1214:refnum<k21>)
            n174 = xnode "FPGA I/O Method Node"("FPGA I/O In"=w1223, "Enable"=w1216) -> ()  [unwired: 1 out]
            n175 = xnode "FPGA I/O Method Node"("FPGA I/O In"=w1222, "Enable"=w1216) -> ()  [unwired: 1 out]
            n176 = xnode "FPGA I/O Method Node"("FPGA I/O In"=w1221, "Enable"=FALSE) -> ()  [unwired: 1 out]
            n177 = xnode "FPGA I/O Node"("I/O Item"=w1211, "FPGA I/O In"=w1212, "I/O Item"=w1211, "FPGA I/O In"=w1215, "I/O Item"=w1211, "FPGA I/O In"=w1214) -> ()  [unwired: 3 out]
            n178 = local write "ADC Init"(FALSE ("ADC Init")) -> ()
          }
        }
      }
      frame #1 {
        # "Message Index"
        # "Channel Index"
        # "16 Bits-Send Channel Selection, CS Normal \n42 Bits Assert Conversion Request, CS Not Enabled\n64 Bits - Unassert Conversion, CS Normal"
        # "CONVERSION REQ"
        n179 = xnode "FPGA I/O Node"("FPGA I/O In"=w1250) -> ("I/O Item"=w1255:bool)  [unwired: 1 out]
        n180 = Bundle By Name(cluster=T7 {"MISO"=FALSE} ("spi input"), "MISO"=w1255) -> (w1256:T7)
        n181 = feedback #14(TRUE ("Chip Select")) -> (w1231:bool)
        n182 = case shown="False" "ADC Manual" {
          tunnel: w1231 -> [w1263 w1316]
          tunnel: [w1263 w1315] -> w1237
          tunnel: [w1268 "ADC SPI Settings"] -> w1236
          tunnel: w1235 -> [w1262 _]
          tunnel: [w1264 "ADC Data In"] -> w1232
          tunnel: [w1261 w1311] -> w1229
          tunnel: [w1267 "ADC Conversion Request"] -> w1233
          tunnel: w1228 -> [w1266 _]
          tunnel: [w1265 w1311] -> w1227
          frame False {
            # "Auto Mode"
            n183 = Boolean To (0,1)(Boolean=w1263) -> (0, 1=w1275:i16)
            n184 = To Unsigned Byte Integer(number=w1275) -> (unsigned 8bit integer=w1274:u8)
            n185 = Add(x=w1274, y=w1262) -> (x+y=w1270:u8)
            n186 = Greater?(x=w1270, y=u8 2) -> (0:w1272:bool)
            n187 = Select(t=u8 0 ("y"), s=w1272, f=w1270) -> (s? t:f=w1269:u8)
            n188 = case shown="1" w1269 {
              selector: w1269 -> [w1282 w1288 w1298]
              tunnel: [w1276 w1285 w1292] -> w1268
              tunnel: [TRUE ("I/O Item") FALSE ("I/O Item") TRUE ("I/O Item")] -> w1267
              tunnel: w1266 -> [w1281 w1289 w1297]
              tunnel: [w1281 w1289 w1296] -> w1265
              tunnel: [w1279 u64 0 u64 53248] -> w1264
              tunnel: w1263 -> [_ _ w1300]
              tunnel: w1262 -> [_ _ w1295]
              tunnel: [w1282 w1288 w1299] -> w1261
              tunnel: "Divide Value" -> [w1277 w1287 w1294]
              frame 0, Default {
                # "16 Bits"
                # "Channel Select"
                # "0x#000"
                n189 = Bundle By Name(cluster=T2 {"Divide Value"=1, "Transfer Length (bits)"=16, "CS Asserted Polarity"=FALSE, "Clock Polarity (CPOL)"=TRUE, "Clock Phase (CPHA)"=FALSE, "Lengthen MISO Setup"=FALSE, "Direction Change Bit"=0, "MOSI Starts as Output"=FALSE, "Tristatable MOSI"=FALSE} ("Master Settings 2"), "Divide Value"=w1277) -> (w1276:T2)
                n190 = To Unsigned Quad Integer(1:w1281) -> (0:w1280:u64)
                n191 = Logical Shift(y=i16 12, x=w1280) -> (x << y=w1279:u64)
              }
              frame 1 {
                # "Conversion Request Asserted"
                # "42 Bits"
                # "Dont Care"
                n192 = Bundle By Name(cluster=T2 {"Divide Value"=1, "Transfer Length (bits)"=42, "CS Asserted Polarity"=FALSE, "Clock Polarity (CPOL)"=TRUE, "Clock Phase (CPHA)"=FALSE, "Lengthen MISO Setup"=FALSE, "Direction Change Bit"=0, "MOSI Starts as Output"=FALSE, "Tristatable MOSI"=FALSE} ("Master Settings 2"), "Divide Value"=w1287) -> (w1285:T2)
              }
              frame 2 {
                # "64 Bits"
                # "Read CMD"
                n193 = Bundle By Name(cluster=T2 {"Divide Value"=1, "Transfer Length (bits)"=64, "CS Asserted Polarity"=FALSE, "Clock Polarity (CPOL)"=TRUE, "Clock Phase (CPHA)"=FALSE, "Lengthen MISO Setup"=FALSE, "Direction Change Bit"=0, "MOSI Starts as Output"=FALSE, "Tristatable MOSI"=FALSE} ("Master Settings 2"), "Divide Value"=w1294) -> (w1292:T2)
                n194 = case shown="False" w1300 {
                  tunnel: [w1303 w1307] -> w1299
                  tunnel: w1298 -> [_ w1307]
                  tunnel: w1297 -> [w1304 w1308]
                  tunnel: [w1304 w1305] -> w1296
                  tunnel: w1295 -> [w1303 _]
                  frame False {
                  }
                  frame True {
                    n195 = Increment(x=w1308) -> (x+1=w1306:u8)
                    n196 = case shown="8" w1306 {
                      selector: w1306 -> [w1309 _]
                      tunnel: [w1309 u8 0] -> w1305
                      frame Default {
                      }
                      frame 8 {
                      }
                    }
                  }
                }
              }
            }
          }
          frame True {
            w1311 = u8 0 ("y")
            # "Manual Mode"
            n197 = feedback #15(FALSE) -> (w1320:bool)
            n198 = feedback-in #15("ADC Trigger") -> ()
            n199 = Greater?(x="ADC Trigger", y=w1320) -> (0:w1317:bool)
            n200 = And(x=w1317, y=w1316) -> (x .and. y?=w1315:bool)
          }
        }
        n201 = call <userlib>:"Spi Master.vi"("spi input"=w1256, "start strobe"=w1237, "data to write"=w1232, "MOSI output enable done"=TRUE, "spi transfer settings"=w1236) -> ("spi output"=w1259:T8, "read data valid"=w1230:bool, "read data"=w1244:u64, "ready for input"=w1246:bool)  [unwired: 7 in]
        "ADC Read Data" <- w1244
        n202 = feedback-in #14(w1246) -> ()
        n203 = Unbundle By Name(w1259) -> ("Chip Select"=w1241:bool, "Clock"=w1245:bool, "MOSI"=w1258:bool)
        n204 = case shown="\"All\", Default" "ADC CS Mode" {
          tunnel: w1241 -> [w1322 w1324 w1328]
          tunnel: [TRUE ("Chip Select") w1324 w1327] -> w1240
          tunnel: [w1322 TRUE ("Chip Select") w1326] -> w1239
          tunnel: w1229 -> [_ _ w1330]
          frame "CS1" {
          }
          frame "CS0" {
          }
          frame "All", Default {
            n205 = Equal?(x=w1330, y=u8 1) -> (x = y?=w1325:bool)
            n206 = case shown="False" w1325 {
              tunnel: w1328 -> [w1331 _]
              tunnel: [w1331 w1332] -> w1327
              tunnel: [w1331 w1332] -> w1326
              frame False {
              }
              frame True {
                w1332 = TRUE ("Chip Select")
              }
            }
          }
        }
        n207 = case shown="True" w1230 {
          tunnel: w1244 -> [_ w1341]
          tunnel: w1254 -> [w1334 w1340]
          tunnel: [w1334 w1339] -> w1253
          tunnel: w1232 -> [_ w1338]
          tunnel: w1227 -> [_ w1337]
          tunnel: w1226 -> [w1333 w1336]
          tunnel: [w1333 w1335] -> w1225
          frame False {
          }
          frame True {
            n208 = case shown="53248" w1338 {
              tunnel: w1341 -> [_ w1372]
              tunnel: w1340 -> [w1343 w1371]
              tunnel: [w1343 w1358] -> w1339
              tunnel: w1337 -> [_ w1364]
              tunnel: w1336 -> [w1342 w1357]
              tunnel: [w1342 w1348] -> w1335
              frame Default {
              }
              frame 53248 {
                w1363 = fxp<+/-,28,17> 0.0 ("AI0")
                # "0xD000"
                n209 = case shown="Default" w1364 {
                  selector: w1364 -> [w1373 _]
                  tunnel: [w1374 u8 7] -> w1365
                  frame Default {
                    n210 = Decrement(x=w1373) -> (x-1=w1374:u8)
                  }
                  frame 0 {
                  }
                }
                n211 = Split Number(x=w1372) -> (hi(x)=w1370:u32, lo(x)=w1369:u32)
                n212 = To Long Integer(number=w1365) -> (32bit integer=w1356:i32)
                n213 = Split Number(x=w1370) -> (hi(x)=w1349:u16, lo(x)=w1351:u16)
                n214 = Split Number(x=w1369) -> (hi(x)=w1352:u16, lo(x)=w1353:u16)
                n215 = To Unsigned Long Integer(number=w1353) -> (unsigned 32bit integer=w1347:u32)
                n216 = To Unsigned Long Integer(number=w1352) -> (unsigned 32bit integer=w1346:u32)
                n217 = To Unsigned Long Integer(number=w1351) -> (unsigned 32bit integer=w1345:u32)
                n218 = To Unsigned Long Integer(number=w1349) -> (unsigned 32bit integer=w1344:u32)
                n219 = To Fixed-Point(fixed-point type=w1363, number=w1349) -> (fixed-point=w1359:fxp<+/-,28,17>)
                n220 = To Fixed-Point(fixed-point type=w1363, number=w1351) -> (fixed-point=w1360:fxp<+/-,28,17>)
                n221 = To Fixed-Point(fixed-point type=w1363, number=w1352) -> (fixed-point=w1361:fxp<+/-,28,17>)
                n222 = To Fixed-Point(fixed-point type=w1363, number=w1353) -> (fixed-point=w1362:fxp<+/-,28,17>)
                n223 = Add(x=w1356, y=8) -> (x+y=w1355:i32)
                n224 = Add(x=w1356, y=16) -> (x+y=w1354:i32)
                n225 = Add(x=w1356, y=24) -> (x+y=w1350:i32)
                n226 = Replace Array Subset(array=w1371, new element #1=w1362, index #1=w1356, new element #2=w1361, index #2=w1355, new element #3=w1360, index #3=w1354, new element #4=w1359, index #4=w1350) -> (w1358:fxp<+/-,28,17>[])
                n227 = Replace Array Subset(array=w1357, new element #1=w1347, index #1=w1356, new element #2=w1346, index #2=w1355, new element #3=w1345, index #3=w1354, new element #4=w1344, index #4=w1350) -> (w1348:u32[])
                n228 = global write "ADC AI Global (U32).vi" "AI16-47 (U32)"(w1348) -> ()
                n229 = global write "ADC AI Global.vi" "AI16-47"(w1358) -> ()
              }
            }
          }
        }
        n230 = xnode "FPGA I/O Node"("I/O Item"=w1239, "FPGA I/O In"=w1248, "I/O Item"=w1240, "FPGA I/O In"=w1249, "I/O Item"=w1245, "FPGA I/O In"=w1252, "I/O Item"=w1258, "FPGA I/O In"=w1251, "I/O Item"=w1233, "FPGA I/O In"=w1234) -> ()  [unwired: 5 out]
      }
    }
  }
  n231 = while {
    shift-right: [w1410] -> _
    shift-left: w3 -> [w1413]
    shift-right: [w1400] -> _
    shift-left: "Initial Acutal Starts" -> [w1407]
    shift-right: [w1411] -> _
    shift-left: w10 -> [w1412]
    shift-right: [w1409] -> _
    shift-left: _ -> [w1408]
    shift-right: [w1398] -> _
    shift-left: "Initial Cmd Starts" -> [w1395]
    shift-right: [w1401] -> _
    shift-left: w5 -> [w1404]
    shift-right: [w1393] -> _
    shift-left: w4 -> [w1394]
    shift-right: [w1392] -> _
    shift-left: w3 -> [w1386]
    shift-right: [w1390] -> _
    shift-left: "Initial No Starts" -> [w1385]
    stop <- FALSE stop-if-true
    # "Pump Current\n(Flange-mount\nCtrl current)"
    n232 = local read "Duty (Ticks)"() -> (w1403:i32[])
    n233 = case shown="True" "Reset Pump Starts" {
      tunnel: w1407 -> [w1417 _]
      tunnel: [w1417 w1418] -> w1405
      tunnel: [w1416 w1418] -> w1396
      tunnel: w1395 -> [w1416 _]
      tunnel: [w1415 w1418] -> w1384
      tunnel: w1385 -> [w1415 _]
      frame False {
      }
      frame True {
        w1418 = u32[] [0, 0, 0, 0, 0, 0] ("Pump Starts")
        n234 = local write "Reset Pump Starts"(FALSE ("Reset Pump Starts")) -> ()
      }
    }
    n235 = global read "Pump Currents Global.vi" "Pump Currents"() -> (w1378:fxp<+/-,28,17>[])
    n236 = Select(t="Ctrl Currents", s="Debug Restarts", f=w1378) -> (s? t:f=w1382:fxp<+/-,28,17>[])
    n237 = for {
      tunnel: w1382 -> [w1424] mode=indexing
      tunnel: w1413 -> [w1451] mode=indexing
      tunnel: w1405 -> [w1450] mode=indexing
      tunnel: [w1449] -> w1400 mode=indexing
      tunnel: w1412 -> [w1447] mode=indexing
      tunnel: [w1448] -> w1411 mode=indexing
      tunnel: [w1446] -> w1410 mode=indexing
      tunnel: [w1445] -> w1409 mode=indexing
      tunnel: w1408 -> [w1444] mode=indexing
      tunnel: w1396 -> [w1438] mode=indexing
      tunnel: w1404 -> [w1442] mode=indexing
      tunnel: w1403 -> [w1439] mode=indexing
      tunnel: "Stop Command" -> [w1443]
      tunnel: [w1437] -> w1398 mode=indexing
      tunnel: [w1439] -> w1401 mode=indexing
      tunnel: w1394 -> [w1433] mode=indexing
      tunnel: [w1430] -> w1393 mode=indexing
      tunnel: [w1434] -> w1392 mode=indexing
      tunnel: w1386 -> [w1432] mode=indexing
      tunnel: "Pump Start Time" -> [w1431]
      tunnel: w1384 -> [w1429] mode=indexing
      tunnel: [w1428] -> w1390 mode=indexing
      tunnel: "Pumps Present" -> [w1422] mode=indexing
      tunnel: "Pump Starts Enable" -> [w1421]
      n238 = And(x=w1422, y=w1421) -> (x .and. y?=w1420:bool)
      n239 = call "Tick Count"() -> ("Tick Count(mSec)"=w1436:u32)
      n240 = Less?(x=w1424, y="Off Current Thresh") -> (x < y?=w1425:bool)
      n241 = Greater?(x=w1424, y="On Current Thresh") -> (0:w1423:bool)
      n242 = Equal?(x=w1443, y=w1442) -> (x = y?=w1441:bool)
      n243 = Not Equal?(x=w1442, y=w1439) -> (x != y?=w1440:bool)
      n244 = Compound Arithmetic op=AND(w1420, w1441, w1440) -> (w1435:bool)
      n245 = case shown="True" w1447 {
        selector: w1447 -> [w1490 w1526]
        tunnel: w1451 -> [w1494 w1530]
        tunnel: w1450 -> [w1493 w1529]
        tunnel: [w1492 w1528] -> w1449
        tunnel: [w1491 w1527] -> w1448
        tunnel: w1436 -> [w1489 w1525]
        tunnel: [w1488 w1524] -> w1446
        tunnel: [w1487 w1523] -> w1445
        tunnel: w1444 -> [w1486 w1522]
        tunnel: w1420 -> [w1485 _]
        tunnel: w1423 -> [w1484 _]
        tunnel: w1425 -> [_ w1521]
        frame False {
          # "Pump is in an off state.  Check\nif it started."
          n246 = case shown="True" w1484 {
            tunnel: w1494 -> [_ w1501]
            tunnel: w1493 -> [w1496 w1507]
            tunnel: [w1496 w1506] -> w1492
            tunnel: w1490 -> [w1498 w1505]
            tunnel: [w1498 w1504] -> w1491
            tunnel: w1489 -> [w1497 w1502]
            tunnel: [w1497 w1503] -> w1488
            tunnel: [w1495 w1500] -> w1487
            tunnel: w1486 -> [w1495 _]
            tunnel: w1485 -> [_ w1499]
            frame False {
              # "Pump is off."
            }
            frame True {
              # "Pump is on, or trying to start."
              n247 = Subtract(x=w1502, y=w1501) -> (x-y=w1500:u32)
              n248 = Greater?(x=w1500, y="Min On Time") -> (0:w1508:bool)
              n249 = case shown="False" w1508 {
                tunnel: w1507 -> [w1512 w1517]
                tunnel: [w1512 w1516] -> w1506
                tunnel: w1505 -> [w1510 _]
                tunnel: [w1510 TRUE] -> w1504
                tunnel: [w1511 w1514] -> w1503
                tunnel: w1502 -> [_ w1514]
                tunnel: w1501 -> [w1511 _]
                tunnel: w1499 -> [_ w1513]
                frame False {
                  # "Pump has NOT met the minimum on time yet."
                }
                frame True {
                  # "Pump has met the minimum on time, so it has started.\nCount this as a successful start."
                  n250 = case shown="True" w1513 {
                    tunnel: w1517 -> [w1518 w1520]
                    tunnel: [w1518 w1519] -> w1516
                    frame False {
                    }
                    frame True {
                      n251 = Increment(x=w1520) -> (x+1=w1519:u32)
                    }
                  }
                }
              }
            }
          }
        }
        frame True {
          # "Pump is in an on state.  Check\nif it stopped."
          n252 = case shown="True" w1521 {
            tunnel: w1530 -> [_ w1536]
            tunnel: w1529 -> [w1533 w1542]
            tunnel: [w1533 w1541] -> w1528
            tunnel: w1526 -> [w1532 w1540]
            tunnel: [w1532 w1539] -> w1527
            tunnel: w1525 -> [w1534 w1537]
            tunnel: [w1534 w1538] -> w1524
            tunnel: [w1531 w1535] -> w1523
            tunnel: w1522 -> [w1531 _]
            frame False {
              # "Pump is in on."
            }
            frame True {
              # "Pump is off, but make sure it's\nacutally off, and not just noise.\nSo, check that current is low\nfor a minimum amount of time."
              n253 = Subtract(x=w1537, y=w1536) -> (x-y=w1535:u32)
              n254 = Greater?(x=w1535, y="Min Off Time") -> (0:w1543:bool)
              n255 = case shown="True" w1543 {
                tunnel: w1542 -> [w1546 w1549]
                tunnel: [w1546 w1549] -> w1541
                tunnel: w1540 -> [w1547 _]
                tunnel: [w1547 FALSE] -> w1539
                tunnel: [w1545 w1548] -> w1538
                tunnel: w1537 -> [_ w1548]
                tunnel: w1536 -> [w1545 _]
                frame False {
                  # "Pump has NOT met the minimum off time yet."
                }
                frame True {
                  # "Pump has met the minimum off time, so it is indeed off."
                }
              }
            }
          }
        }
      }
      n256 = case shown="True" w1433 {
        selector: w1433 -> [_ w1458]
        tunnel: w1438 -> [w1455 w1457]
        tunnel: [w1455 w1456] -> w1437
        tunnel: w1436 -> [w1454 w1464]
        tunnel: w1435 -> [w1453 _]
        tunnel: [w1454 w1465] -> w1434
        tunnel: w1432 -> [_ w1459]
        tunnel: w1431 -> [_ w1468]
        tunnel: [w1453 w1463] -> w1430
        tunnel: w1429 -> [w1452 w1467]
        tunnel: [w1452 w1466] -> w1428
        tunnel: w1423 -> [_ w1460]
        frame False {
        }
        frame True {
          n257 = Subtract(x=w1464, y=w1459) -> (x-y=w1469:u32)
          n258 = Greater?(x=w1469, y=w1468) -> (0:w1462:bool)
          n259 = Or(x=w1460, y=w1462) -> (x .or. y?=w1461:bool)
          n260 = case shown="True" w1461 {
            tunnel: w1467 -> [w1471 w1480]
            tunnel: [w1471 w1479] -> w1466
            tunnel: [w1473 w1478] -> w1465
            tunnel: w1464 -> [_ w1478]
            tunnel: [w1472 FALSE] -> w1463
            tunnel: w1460 -> [_ w1476]
            tunnel: w1459 -> [w1473 _]
            tunnel: w1458 -> [w1472 _]
            tunnel: w1457 -> [w1470 w1475]
            tunnel: [w1470 w1474] -> w1456
            frame False {
            }
            frame True {
              n261 = case shown="False" w1476 {
                tunnel: w1480 -> [w1482 w1483]
                tunnel: [w1481 w1483] -> w1479
                frame False {
                  n262 = Increment(x=w1482) -> (x+1=w1481:u32)
                }
                frame True {
                }
              }
              n263 = Increment(x=w1475) -> (x+1=w1474:u32)
            }
          }
        }
      }
    }
    "Actual Pump Starts" <- w1400
    "Timers (ms)" <- w1409
    "Pump On States" <- w1411
    "Cmd Pump Starts" <- w1398
    "Pump No Starts" <- w1390
    n264 = To Long Integer(number=w1400) -> (32bit integer=w1399:i32[])
    n265 = To Long Integer(number=w1398) -> (32bit integer=w1397:i32[])
    n266 = To Long Integer(number=w1390) -> (32bit integer=w1388:i32[])
    n267 = Subtract(x=w1399, y=w1397) -> (x-y=w1389:i32[])
    n268 = Add(x=w1389, y=w1388) -> (x+y=→"Restarts":i32[])
  }
  n269 = timed-loop "AI Resample Loop" {
    timing: w51 -> [_]
    timing-out: [_] -> w50
    shift-right: [w1573] -> _
    shift-left: u32 0 ("Sample Divisor") -> [w1560]
    shift-right: [w1572] -> _
    shift-left: w47 -> [w1561]
    tunnel: w48 -> [w1566]
    tunnel: w47 -> [w1565]
    stop <- FALSE stop-if-true
    # "Press, Flow"
    # "Ctrlr Current"
    # "30 items"
    n270 = global read "ADC AI Global (U32).vi" "AI16-47 (U32)"() -> (w1554:u32[])
    n271 = local read "Actual Pump Starts"() -> (w1551:u32[])
    n272 = global read "Diagnostic Global (U32).vi" "Diag Global (U32)"() -> (w1552:u32[])
    n273 = Less Or Equal?(x="AI Divisor", y=w1560) -> (x <= y?=w1564:bool)
    n274 = Array Subset(array=w1554, length=6) -> (w1556:u32[])  [unwired: 1 in]
    n275 = Array Subset(array=w1554, index=14, length=6) -> (w1555:u32[])
    n276 = Build Array (concatenate)(w1556, w1555, w1551, w1552, "Pump Cmds (Duty)") -> (w1562:u32[])
    n277 = feedback #16() -> (w1568:u32[])  [unwired: 1 in]
    n278 = Select(t=w1562, s=w1564, f=w1568) -> (s? t:f=w1567:u32[])
    n279 = feedback-in #16(w1567) -> ()
    n280 = Less Or Equal?(x=w1561, y=w1566) -> (x <= y?=w1570:bool)
    n281 = Or(x=w1564, y=w1570) -> (x .or. y?=w1563:bool)
    n282 = case shown="True" w1563 {
      tunnel: w1561 -> [_ w1582]
      tunnel: [w1580 w1583] -> w1569
      tunnel: w1567 -> [_ w1581]
      tunnel: w1565 -> [w1580 _]
      frame False {
      }
      frame True {
        n283 = Decrement(x=w1582) -> (x-1=w1583:u8)
        n284 = case shown="Default" w1583 {
          selector: w1583 -> [w1590 _ _]
          tunnel: [w1588 u32 4294967295 ("AI0") u32 0 ("AI0")] -> w1585
          tunnel: [TRUE TRUE FALSE] -> w1584
          tunnel: w1581 -> [w1592 _ _]
          frame 1..30 {
            # "Data case for\nAI Data"
            n285 = Subtract(x=u8 30 ("Sample Divisor"), y=w1590) -> (x-y=w1589:u8)
            n286 = Index Array(array=w1592, index=w1589) -> (element=w1588:u32)
          }
          frame 0 {
            # "Used to write AI Data\nIndexer"
          }
          frame Default {
            # "Sould never get to\nthis case."
          }
        }
        n287 = case shown="True" w1584 {
          tunnel: w1585 -> [_ w1587]
          frame False {
          }
          frame True {
            n288 = xnode ("FIFO Method Node")("Element"=w1587, "Timeout"=u8 0) -> ()  [unwired: 1 in, 2 out]
          }
        }
      }
    }
    n289 = case shown="False" w1564 {
      tunnel: w1560 -> [w1577 _]
      tunnel: [w1576 u32 0] -> w1573
      tunnel: w1569 -> [w1575 w1578]
      tunnel: [w1575 w1578] -> w1572
      frame False {
        n290 = Increment(x=w1577) -> (x+1=w1576:u32)
      }
      frame True {
      }
    }
  }
  n291 = timed-loop {
    timing: w12 -> [_]
    timing-out: [_] -> w11
    stop <- FALSE stop-if-true
    (unwired) fxp<+/-,28,17>[] [0.0, 0.0, 0.0, 0.0, 0.0, 0.0]  # Speed Placeholder
    n292 = global read "Pump Currents Global.vi" "Pump Currents"() -> (w1605:fxp<+/-,28,17>[])
    n293 = global read "ADC AI Global (Avg).vi" "AI22-47 (Avg)"() -> (w1604:fxp<+/-,28,17>[])
    n294 = local read "Elapsed Times"() -> (→"Elapsed Times OUT":fxp<+,40,40>[])
    n295 = global read "Onboard AIs Global.vi" "Onboard AI's"() -> (w1603:fxp<+/-,28,17>[])
    n296 = global read "Diagnostic Global.vi" "Diag_Global"() -> (w1606:fxp<+/-,28,17>[])
    n297 = local read "Pump Cmds"() -> (w1600:fxp<+/-,28,17>[])
    n298 = Build Array (concatenate)(w1603, w1605, w1600, w1604, w1606) -> (→"Data OUT":fxp<+/-,28,17>[])
  }
  n299 = node-c288(w31) -> ()
  n300 = while {
    stop <- FALSE stop-if-true
    n301 = xnode "FPGA I/O Node"("AO0"="PS Cmd", "AO1"="Pressure Cmd", "AO2"="AO2", "AO3"="AO3") -> ()  [unwired: 5 in, 5 out]
  }
  n302 = while {
    stop <- FALSE stop-if-true
    w1622 = fxp<+/-,28,17> 0.0 ("Controller_Current_1 (AI6)")
    # "set at 100 Hz"
    # "S 28 17"
    # "S 24 5"
    n303 = xnode "FPGA I/O Node"() -> ("Voltage_1 (AI0/8)"=w1628:fxp<+/-,24,5>, "Voltage_2 (AI1/9)"=w1624:fxp<+/-,24,5>, "Voltage_3 (AI2/10)"=w1625:fxp<+/-,24,5>, "Voltage_4 (AI3/11)"=w1623:fxp<+/-,24,5>, "Voltage_5 (AI4/12)"=w1626:fxp<+/-,24,5>, "Voltage_6 (AI5/13)"=w1627:fxp<+/-,24,5>, "Spare_1"=w1635:fxp<+/-,24,5>, "Spare_2"=w1636:fxp<+/-,24,5>, "Spare_3"=w1637:fxp<+/-,24,5>, "PS_Sense (AI15)"=w1638:fxp<+/-,24,5>)  [unwired: 10 in, 10 out]
    n304 = To Fixed-Point(fixed-point type=w1622, number=w1628) -> (fixed-point=w1621:fxp<+/-,28,17>)
    n305 = To Fixed-Point(fixed-point type=w1622, number=w1624) -> (fixed-point=w1620:fxp<+/-,28,17>)
    n306 = To Fixed-Point(fixed-point type=w1622, number=w1625) -> (fixed-point=w1619:fxp<+/-,28,17>)
    n307 = To Fixed-Point(fixed-point type=w1622, number=w1623) -> (fixed-point=w1617:fxp<+/-,28,17>)
    n308 = To Fixed-Point(fixed-point type=w1622, number=w1626) -> (fixed-point=w1616:fxp<+/-,28,17>)
    n309 = To Fixed-Point(fixed-point type=w1622, number=w1627) -> (fixed-point=w1615:fxp<+/-,28,17>)
    n310 = To Fixed-Point(fixed-point type=w1622, number=w1635) -> (fixed-point=w1630:fxp<+/-,28,17>)
    n311 = To Fixed-Point(fixed-point type=w1622, number=w1636) -> (fixed-point=w1631:fxp<+/-,28,17>)
    n312 = To Fixed-Point(fixed-point type=w1622, number=w1637) -> (fixed-point=w1632:fxp<+/-,28,17>)
    n313 = To Fixed-Point(fixed-point type=w1622, number=w1638) -> (fixed-point=w1633:fxp<+/-,28,17>)
    n314 = Build Array(w1621, w1620, w1619, w1617, w1616, w1615, w1630, w1631, w1632, w1633) -> (w1618:fxp<+/-,28,17>[])
    n315 = global write "Onboard AIs Global.vi" "Onboard AI's"(w1618) -> ()
    n316 = call "Wait"("Count(mSec)"=u32 10) -> ()  [unwired: 1 out]
  }
  n317 = node-c288(w11) -> ()
  n318 = while {
    shift-right: [w1649] -> _
    shift-left: 0 ("Moving Point Index") -> [w1650]
    stop <- FALSE stop-if-true
    w1648 = 127 ("N (# of Ave Pts 8 max)")
    # "Ctrl Current, Temp,\nPressure, Flow\nAI22-47"
    # "S 28 17"
    # "set at 1 kHz"
    n319 = global read "Flow Frequencies Global.vi" "Flow Frequencies"() -> (w1639:fxp<+/-,28,17>[])
    n320 = global read "ADC AI Global.vi" "AI16-47"() -> (w1644:fxp<+/-,28,17>[])
    n321 = Array Subset(array=w1644, index=6, length=26) -> (w1641:fxp<+/-,28,17>[])
    n322 = case shown="True" "Freq Flow?" {
      tunnel: w1641 -> [w1656 w1660]
      tunnel: w1639 -> [_ w1659]
      tunnel: [w1656 w1657] -> w1640
      frame False {
      }
      frame True {
        n323 = Replace Array Subset(array=w1660, new element=w1659, index=14) -> (w1657:fxp<+/-,28,17>[])
      }
    }
    n324 = for {
      tunnel: w1650 -> [w1661]
      tunnel: w1648 -> [w1662]
      tunnel: [w1666] -> w1643 mode=indexing
      tunnel: w1640 -> [w1665] mode=indexing
      tunnel: refnum<k21> "Running Avg Memory" ("Memory") -> [w1664]
      i -> [w1663]
      n325 = call "Moving Average.vi"("Memory In"=w1664, "N (# of Ave Pts 127 max)"=w1662, "Moving Point Index"=w1661, "Data IN"=w1665, "Channel#"=w1663) -> ("Averaged Data"=w1666:fxp<+/-,28,17>)  [unwired: 10 in]
    }
    n326 = global write "ADC AI Global (Avg).vi" "AI22-47 (Avg)"(w1643) -> ()
    n327 = Increment(x=w1650) -> (x+1=w1652:i32)
    n328 = Greater Or Equal?(x=w1650, y=w1648) -> (x >= y?=w1651:bool)
    n329 = Select(t=0, s=w1651, f=w1652) -> (s? t:f=w1649:i32)
    n330 = call "Wait2"("Count(mSec)"=u32 1) -> ()  [unwired: 1 out]
  }
  n331 = while {
    stop <- FALSE stop-if-true
    n332 = local read "Pump Cmds (Duty)"() -> (w1668:u32[])
    n333 = for {
      tunnel: w1668 -> [w1671] mode=indexing
      tunnel: [w1670] -> w1667 mode=indexing
      n334 = To Fixed-Point(fixed-point type=fxp<+/-,28,17> 0.0 ("AI0"), number=w1671) -> (fixed-point=w1670:fxp<+/-,28,17>)
    }
    "Pump Cmds" <- w1667
  }
  n335 = node-c288(w29) -> ()
  n336 = node-c288() -> (w14:T4)  [unwired: 1 in]
  n337 = timed-loop {
    shift-right: [w1752] -> _
    shift-left: _ -> [w1751]
    shift-right: [w1750] -> _
    shift-left: _ -> [w1749]
    shift-right: [w1747] -> _
    shift-left: _ -> [w1748]
    shift-right: [w1745] -> _
    shift-left: _ -> [w1746]
    timing: w14 -> [_]
    timing-out: [_] -> w13
    shift-right: [w1743] -> _
    shift-left: _ -> [w1744]
    shift-right: [w1734] -> _
    shift-left: _ -> [w1735]
    shift-right: [w1736] -> _
    shift-left: _ -> [w1737]
    shift-right: [w1739] -> _
    shift-left: _ -> [w1738]
    shift-right: [w1741] -> _
    shift-left: _ -> [w1740]
    shift-right: [w1697] -> _
    shift-left: _ -> [w1742]
    shift-right: [w1733] -> _
    shift-left: _ -> [w1732]
    shift-right: [w1731] -> _
    shift-left: _ -> [w1730]
    shift-right: [w1728] -> _
    shift-left: _ -> [w1729]
    shift-right: [w1726] -> _
    shift-left: _ -> [w1727]
    shift-right: [w1696] -> _
    shift-left: _ -> [w1725]
    shift-right: [w1716] -> _
    shift-left: _ -> [w1717]
    shift-right: [w1718] -> _
    shift-left: _ -> [w1719]
    shift-right: [w1721] -> _
    shift-left: _ -> [w1720]
    shift-right: [w1723] -> _
    shift-left: _ -> [w1722]
    shift-right: [w1695] -> _
    shift-left: _ -> [w1724]
    shift-right: [w1715] -> _
    shift-left: _ -> [w1714]
    shift-right: [w1713] -> _
    shift-left: _ -> [w1712]
    shift-right: [w1710] -> _
    shift-left: _ -> [w1711]
    shift-right: [w1708] -> _
    shift-left: _ -> [w1709]
    shift-right: [w1694] -> _
    shift-left: _ -> [w1707]
    shift-right: [w1698] -> _
    shift-left: _ -> [w1699]
    shift-right: [w1700] -> _
    shift-left: _ -> [w1701]
    shift-right: [w1703] -> _
    shift-left: _ -> [w1702]
    shift-right: [w1705] -> _
    shift-left: _ -> [w1704]
    shift-right: [w1693] -> _
    shift-left: _ -> [w1706]
    stop <- FALSE stop-if-true
    n338 = xnode "FPGA I/O Node"() -> ("RMC/DIO38"=w1673:bool)  [unwired: 1 in, 1 out]
    n339 = xnode "FPGA I/O Node"() -> ("RMC/DIO39"=w1691:bool)  [unwired: 1 in, 1 out]
    n340 = xnode "FPGA I/O Node"() -> ("RMC/DIO40"=w1689:bool)  [unwired: 1 in, 1 out]
    n341 = xnode "FPGA I/O Node"() -> ("RMC/DIO41"=w1687:bool)  [unwired: 1 in, 1 out]
    n342 = xnode "FPGA I/O Node"() -> ("RMC/DIO42"=w1685:bool)  [unwired: 1 in, 1 out]
    n343 = xnode "FPGA I/O Node"() -> ("RMC/DIO43"=w1683:bool)  [unwired: 1 in, 1 out]
    n344 = call "FPGA Debounce Digital.vi"("Input Signal"=w1673, "Cycles to Filter"="Diagnostic Filter") -> ("Output Filtered Signal"=w1692:bool)
    n345 = call "FPGA Debounce Digital.vi"("Input Signal"=w1691, "Cycles to Filter"="Diagnostic Filter") -> ("Output Filtered Signal"=w1690:bool)
    n346 = call "FPGA Debounce Digital.vi"("Input Signal"=w1689, "Cycles to Filter"="Diagnostic Filter") -> ("Output Filtered Signal"=w1688:bool)
    n347 = call "FPGA Debounce Digital.vi"("Input Signal"=w1687, "Cycles to Filter"="Diagnostic Filter") -> ("Output Filtered Signal"=w1686:bool)
    n348 = call "FPGA Debounce Digital.vi"("Input Signal"=w1685, "Cycles to Filter"="Diagnostic Filter") -> ("Output Filtered Signal"=w1684:bool)
    n349 = call "FPGA Debounce Digital.vi"("Input Signal"=w1683, "Cycles to Filter"="Diagnostic Filter") -> ("Output Filtered Signal"=w1682:bool)
    n350 = To Fixed-Point(fixed-point type=fxp<+/-,32,32> 0.0 ("s? t:f"), number="Diagnostic Freq Coeff") -> (fixed-point=w1679:fxp<+/-,32,32>)
    n351 = case shown="\"CMFB\"" "Diagnostic Mode" {
      tunnel: [w1756 w1899 w2226] -> w1752
      tunnel: w1751 -> [_ w1898 w2227]
      tunnel: [w1754 w1897 w2122] -> w1750
      tunnel: w1749 -> [_ w1896 _]
      tunnel: w1748 -> [_ w1895 _]
      tunnel: [w1756 w1889 w2123] -> w1747
      tunnel: w1746 -> [_ w1888 _]
      tunnel: [w1756 w1887 w2123] -> w1745
      tunnel: w1744 -> [_ w1883 w2228]
      tunnel: [w1755 w1882 w2121] -> w1743
      tunnel: w1742 -> [_ w1881 w2143]
      tunnel: [w1756 w1877 w2123] -> w1741
      tunnel: w1740 -> [_ w1876 _]
      tunnel: [w1756 w1875 w2123] -> w1739
      tunnel: w1738 -> [_ w1869 _]
      tunnel: w1737 -> [_ w1868 _]
      tunnel: [w1754 w1867 w2122] -> w1736
      tunnel: w1735 -> [_ w1866 w2144]
      tunnel: [w1756 w1865 w2142] -> w1734
      tunnel: [w1756 w1854 w2138] -> w1733
      tunnel: w1732 -> [_ w1853 w2140]
      tunnel: [w1754 w1852 w2122] -> w1731
      tunnel: w1730 -> [_ w1851 _]
      tunnel: w1729 -> [_ w1850 _]
      tunnel: [w1756 w1844 w2123] -> w1728
      tunnel: w1727 -> [_ w1843 _]
      tunnel: [w1756 w1842 w2123] -> w1726
      tunnel: w1725 -> [_ w1838 w2139]
      tunnel: w1724 -> [_ w1837 w2136]
      tunnel: [w1756 w1833 w2123] -> w1723
      tunnel: w1722 -> [_ w1832 _]
      tunnel: [w1756 w1831 w2123] -> w1721
      tunnel: w1720 -> [_ w1825 _]
      tunnel: w1719 -> [_ w1824 _]
      tunnel: [w1754 w1823 w2122] -> w1718
      tunnel: w1717 -> [_ w1822 w2134]
      tunnel: [w1756 w1821 w2135] -> w1716
      tunnel: [w1756 w1810 w2130] -> w1715
      tunnel: w1714 -> [_ w1809 w2132]
      tunnel: [w1754 w1808 w2122] -> w1713
      tunnel: w1712 -> [_ w1807 _]
      tunnel: w1711 -> [_ w1806 _]
      tunnel: [w1756 w1800 w2123] -> w1710
      tunnel: w1709 -> [_ w1799 _]
      tunnel: [w1756 w1798 w2123] -> w1708
      tunnel: w1707 -> [_ w1794 w2131]
      tunnel: w1706 -> [_ w1793 w2125]
      tunnel: [w1756 w1789 w2123] -> w1705
      tunnel: w1704 -> [_ w1788 _]
      tunnel: [w1756 w1787 w2123] -> w1703
      tunnel: w1702 -> [_ w1781 _]
      tunnel: w1701 -> [_ w1780 _]
      tunnel: [w1754 w1779 w2122] -> w1700
      tunnel: w1699 -> [_ w1778 w2126]
      tunnel: [w1756 w1777 w2124] -> w1698
      tunnel: [w1755 w1771 w2120] -> w1697
      tunnel: [w1755 w1770 w2119] -> w1696
      tunnel: [w1755 w1769 w2118] -> w1695
      tunnel: [w1755 w1768 w2117] -> w1694
      tunnel: [w1755 w1767 w2116] -> w1693
      tunnel: w1692 -> [_ w1766 w2229]
      tunnel: w1690 -> [_ w1765 w2145]
      tunnel: w1688 -> [_ w1764 w2141]
      tunnel: w1686 -> [_ w1763 w2137]
      tunnel: w1684 -> [_ w1762 w2133]
      tunnel: w1682 -> [_ w1761 w2127]
      tunnel: w1679 -> [_ w1760 _]
      tunnel: "Invert Diagnostic" -> [_ w1759 _]
      tunnel: "Diag Max Period (ticks)" -> [_ _ w2128]
      tunnel: [fxp<+/-,28,17>[] [0.0, 0.0, 0.0, 0.0, 0.0, 0.0] w1758 w2115] -> w1674
      frame "None", Default {
        w1754 = FALSE ("Output Filtered Signal")
        w1755 = fxp<+/-,28,17> 0.0 ("AI0")
        w1756 = u32 0 ("f")
      }
      frame "PSA" {
        # "PWM diagnostic code."
        n352 = call "Tick Count2"() -> ("Tick Count(Ticks)"=w1904:u32)
        n353 = call "Tick Count3"() -> ("Tick Count(Ticks)"=w1860:u32)
        n354 = call "Tick Count4"() -> ("Tick Count(Ticks)"=w1859:u32)
        n355 = call "Tick Count5"() -> ("Tick Count(Ticks)"=w1816:u32)
        n356 = call "Tick Count6"() -> ("Tick Count(Ticks)"=w1815:u32)
        n357 = call "Tick Count7"() -> ("Tick Count(Ticks)"=w1772:u32)
        n358 = Greater?(x=w1766, y=w1896) -> (0:w1901:bool)
        n359 = Greater?(x=w1765, y=w1868) -> (0:w1863:bool)
        n360 = Greater?(x=w1764, y=w1851) -> (0:w1856:bool)
        n361 = Greater?(x=w1763, y=w1824) -> (0:w1819:bool)
        n362 = Greater?(x=w1762, y=w1807) -> (0:w1812:bool)
        n363 = Greater?(x=w1761, y=w1780) -> (0:w1775:bool)
        n364 = Subtract(x=w1904, y=w1898) -> (x-y=w1903:u32)
        n365 = Subtract(x=w1860, y=w1866) -> (x-y=w1861:u32)
        n366 = Subtract(x=w1859, y=w1853) -> (x-y=w1858:u32)
        n367 = Subtract(x=w1816, y=w1822) -> (x-y=w1817:u32)
        n368 = Subtract(x=w1815, y=w1809) -> (x-y=w1814:u32)
        n369 = Subtract(x=w1772, y=w1778) -> (x-y=w1773:u32)
        n370 = Less?(x=w1766, y=w1896) -> (x < y?=w1902:bool)
        n371 = Less?(x=w1765, y=w1868) -> (x < y?=w1862:bool)
        n372 = Less?(x=w1764, y=w1851) -> (x < y?=w1857:bool)
        n373 = Less?(x=w1763, y=w1824) -> (x < y?=w1818:bool)
        n374 = Less?(x=w1762, y=w1807) -> (x < y?=w1813:bool)
        n375 = Less?(x=w1761, y=w1780) -> (x < y?=w1774:bool)
        n376 = case shown="True" w1759 {
          tunnel: w1902 -> [w2111 w2113]
          tunnel: w1901 -> [w2110 w2114]
          tunnel: [w2111 w2114] -> w1900
          tunnel: [w2110 w2113] -> w1886
          tunnel: w1766 -> [w2109 w2112]
          tunnel: [w2109 w2112] -> w1897
          frame False {
          }
          frame True {
          }
        }
        n377 = case shown="True" w1759 {
          tunnel: w1862 -> [w2076 w2078]
          tunnel: w1863 -> [w2075 w2079]
          tunnel: [w2076 w2079] -> w1864
          tunnel: [w2075 w2078] -> w1878
          tunnel: w1765 -> [w2074 w2077]
          tunnel: [w2074 w2077] -> w1867
          frame False {
          }
          frame True {
          }
        }
        n378 = case shown="True" w1759 {
          tunnel: w1857 -> [w2041 w2043]
          tunnel: w1856 -> [w2040 w2044]
          tunnel: [w2041 w2044] -> w1855
          tunnel: [w2040 w2043] -> w1841
          tunnel: w1764 -> [w2039 w2042]
          tunnel: [w2039 w2042] -> w1852
          frame False {
          }
          frame True {
          }
        }
        n379 = case shown="True" w1759 {
          tunnel: w1818 -> [w2006 w2008]
          tunnel: w1819 -> [w2005 w2009]
          tunnel: [w2006 w2009] -> w1820
          tunnel: [w2005 w2008] -> w1834
          tunnel: w1763 -> [w2004 w2007]
          tunnel: [w2004 w2007] -> w1823
          frame False {
          }
          frame True {
          }
        }
        n380 = case shown="True" w1759 {
          tunnel: w1813 -> [w1971 w1973]
          tunnel: w1812 -> [w1970 w1974]
          tunnel: [w1971 w1974] -> w1811
          tunnel: [w1970 w1973] -> w1797
          tunnel: w1762 -> [w1969 w1972]
          tunnel: [w1969 w1972] -> w1808
          frame False {
          }
          frame True {
          }
        }
        n381 = case shown="True" w1759 {
          tunnel: w1774 -> [w1936 w1938]
          tunnel: w1775 -> [w1935 w1939]
          tunnel: [w1936 w1939] -> w1776
          tunnel: [w1935 w1938] -> w1790
          tunnel: w1761 -> [w1934 w1937]
          tunnel: [w1934 w1937] -> w1779
          frame False {
          }
          frame True {
          }
        }
        n382 = Select(t=w1903, s=w1900, f=w1895) -> (s? t:f=w1889:u32)
        n383 = Select(t=w1861, s=w1864, f=w1869) -> (s? t:f=w1875:u32)
        n384 = Select(t=w1858, s=w1855, f=w1850) -> (s? t:f=w1844:u32)
        n385 = Select(t=w1817, s=w1820, f=w1825) -> (s? t:f=w1831:u32)
        n386 = Select(t=w1814, s=w1811, f=w1806) -> (s? t:f=w1800:u32)
        n387 = Select(t=w1773, s=w1776, f=w1781) -> (s? t:f=w1787:u32)
        n388 = Select(t=w1904, s=w1886, f=w1898) -> (s? t:f=w1899:u32)
        n389 = Select(t=w1860, s=w1878, f=w1866) -> (s? t:f=w1865:u32)
        n390 = Select(t=w1859, s=w1841, f=w1853) -> (s? t:f=w1854:u32)
        n391 = Select(t=w1816, s=w1834, f=w1822) -> (s? t:f=w1821:u32)
        n392 = Select(t=w1815, s=w1797, f=w1809) -> (s? t:f=w1810:u32)
        n393 = Select(t=w1772, s=w1790, f=w1778) -> (s? t:f=w1777:u32)
        n394 = Select(t=w1889, s=w1886, f=w1888) -> (s? t:f=w1887:u32)
        n395 = Select(t=w1875, s=w1878, f=w1876) -> (s? t:f=w1877:u32)
        n396 = Select(t=w1844, s=w1841, f=w1843) -> (s? t:f=w1842:u32)
        n397 = Select(t=w1831, s=w1834, f=w1832) -> (s? t:f=w1833:u32)
        n398 = Select(t=w1800, s=w1797, f=w1799) -> (s? t:f=w1798:u32)
        n399 = Select(t=w1787, s=w1790, f=w1788) -> (s? t:f=w1789:u32)
        n400 = To Fixed-Point(fixed-point type=fxp<+/-,32,32> 0.0 ("s? t:f"), number=w1887) -> (fixed-point=w1890:fxp<+/-,32,32>)
        n401 = To Fixed-Point(fixed-point type=fxp<+/-,32,32> 0.0 ("s? t:f"), number=w1877) -> (fixed-point=w1874:fxp<+/-,32,32>)
        n402 = To Fixed-Point(fixed-point type=fxp<+/-,32,32> 0.0 ("s? t:f"), number=w1842) -> (fixed-point=w1845:fxp<+/-,32,32>)
        n403 = To Fixed-Point(fixed-point type=fxp<+/-,32,32> 0.0 ("s? t:f"), number=w1833) -> (fixed-point=w1830:fxp<+/-,32,32>)
        n404 = To Fixed-Point(fixed-point type=fxp<+/-,32,32> 0.0 ("s? t:f"), number=w1798) -> (fixed-point=w1801:fxp<+/-,32,32>)
        n405 = To Fixed-Point(fixed-point type=fxp<+/-,32,32> 0.0 ("s? t:f"), number=w1789) -> (fixed-point=w1786:fxp<+/-,32,32>)
        n406 = feedback #17() -> (w1891:bool)  [unwired: 1 in]
        n407 = And(x=w1886, y=w1891) -> (x .and. y?=w1892:bool)
        n408 = feedback #18() -> (w1873:bool)  [unwired: 1 in]
        n409 = And(x=w1878, y=w1873) -> (x .and. y?=w1872:bool)
        n410 = feedback #19() -> (w1846:bool)  [unwired: 1 in]
        n411 = And(x=w1841, y=w1846) -> (x .and. y?=w1847:bool)
        n412 = feedback #20() -> (w1829:bool)  [unwired: 1 in]
        n413 = And(x=w1834, y=w1829) -> (x .and. y?=w1828:bool)
        n414 = feedback #21() -> (w1802:bool)  [unwired: 1 in]
        n415 = And(x=w1797, y=w1802) -> (x .and. y?=w1803:bool)
        n416 = feedback #22() -> (w1785:bool)  [unwired: 1 in]
        n417 = And(x=w1790, y=w1785) -> (x .and. y?=w1784:bool)
        n418 = xnode "High Throughput Divide"("x"=w1890, "y"=w1760, "input valid"=w1892) -> ("x/y"=w1885:fxp<+/-,28,17>, "output valid"=w1884:bool, "ready for input"=w1893:bool)  [unwired: 1 in]
        n419 = feedback-in #17(w1893) -> ()
        n420 = xnode "High Throughput Divide"("x"=w1874, "y"=w1760, "input valid"=w1872) -> ("x/y"=w1879:fxp<+/-,28,17>, "output valid"=w1880:bool, "ready for input"=w1871:bool)  [unwired: 1 in]
        n421 = feedback-in #18(w1871) -> ()
        n422 = xnode "High Throughput Divide"("x"=w1845, "y"=w1760, "input valid"=w1847) -> ("x/y"=w1840:fxp<+/-,28,17>, "output valid"=w1839:bool, "ready for input"=w1848:bool)  [unwired: 1 in]
        n423 = feedback-in #19(w1848) -> ()
        n424 = xnode "High Throughput Divide"("x"=w1830, "y"=w1760, "input valid"=w1828) -> ("x/y"=w1835:fxp<+/-,28,17>, "output valid"=w1836:bool, "ready for input"=w1827:bool)  [unwired: 1 in]
        n425 = feedback-in #20(w1827) -> ()
        n426 = xnode "High Throughput Divide"("x"=w1801, "y"=w1760, "input valid"=w1803) -> ("x/y"=w1796:fxp<+/-,28,17>, "output valid"=w1795:bool, "ready for input"=w1804:bool)  [unwired: 1 in]
        n427 = feedback-in #21(w1804) -> ()
        n428 = xnode "High Throughput Divide"("x"=w1786, "y"=w1760, "input valid"=w1784) -> ("x/y"=w1791:fxp<+/-,28,17>, "output valid"=w1792:bool, "ready for input"=w1783:bool)  [unwired: 1 in]
        n429 = feedback-in #22(w1783) -> ()
        n430 = Select(t=w1885, s=w1884, f=w1883) -> (s? t:f=w1882:fxp<+/-,28,17>)
        n431 = Select(t=w1879, s=w1880, f=w1881) -> (s? t:f=w1771:fxp<+/-,28,17>)
        n432 = Select(t=w1840, s=w1839, f=w1838) -> (s? t:f=w1770:fxp<+/-,28,17>)
        n433 = Select(t=w1835, s=w1836, f=w1837) -> (s? t:f=w1769:fxp<+/-,28,17>)
        n434 = Select(t=w1796, s=w1795, f=w1794) -> (s? t:f=w1768:fxp<+/-,28,17>)
        n435 = Select(t=w1791, s=w1792, f=w1793) -> (s? t:f=w1767:fxp<+/-,28,17>)
        n436 = Build Array(w1882, w1771, w1770, w1769, w1768, w1767) -> (w1758:fxp<+/-,28,17>[])
      }
      frame "CMFB" {
        w2122 = FALSE ("Output Filtered Signal")
        w2123 = u32 0
        w2129 = fxp<+,32,32> 40000000.0 ("x")
        # "CMFB diagnostic code."
        n437 = feedback #23() -> (w2245:bool)  [unwired: 1 in]
        n438 = feedback-in #23(w2229) -> ()
        n439 = feedback #24() -> (w2210:bool)  [unwired: 1 in]
        n440 = feedback-in #24(w2145) -> ()
        n441 = feedback #25() -> (w2209:bool)  [unwired: 1 in]
        n442 = feedback-in #25(w2141) -> ()
        n443 = feedback #26() -> (w2178:bool)  [unwired: 1 in]
        n444 = feedback-in #26(w2137) -> ()
        n445 = feedback #27() -> (w2177:bool)  [unwired: 1 in]
        n446 = feedback-in #27(w2133) -> ()
        n447 = feedback #28() -> (w2146:bool)  [unwired: 1 in]
        n448 = feedback-in #28(w2127) -> ()
        n449 = Increment(x=w2227) -> (x+1=w2242:u32)
        n450 = Increment(x=w2144) -> (x+1=w2213:u32)
        n451 = Increment(x=w2140) -> (x+1=w2206:u32)
        n452 = Increment(x=w2134) -> (x+1=w2181:u32)
        n453 = Increment(x=w2132) -> (x+1=w2174:u32)
        n454 = Increment(x=w2126) -> (x+1=w2149:u32)
        n455 = Greater?(x=w2229, y=w2245) -> (0:w2230:bool)
        n456 = Greater?(x=w2145, y=w2210) -> (0:w2225:bool)
        n457 = Greater?(x=w2141, y=w2209) -> (0:w2194:bool)
        n458 = Greater?(x=w2137, y=w2178) -> (0:w2193:bool)
        n459 = Greater?(x=w2133, y=w2177) -> (0:w2162:bool)
        n460 = Greater?(x=w2127, y=w2146) -> (0:w2161:bool)
        n461 = Greater?(x=w2242, y=w2128) -> (0:w2244:bool)
        n462 = Greater?(x=w2213, y=w2128) -> (0:w2211:bool)
        n463 = Greater?(x=w2206, y=w2128) -> (0:w2208:bool)
        n464 = Greater?(x=w2181, y=w2128) -> (0:w2179:bool)
        n465 = Greater?(x=w2174, y=w2128) -> (0:w2176:bool)
        n466 = Greater?(x=w2149, y=w2128) -> (0:w2147:bool)
        n467 = To Fixed-Point(number=w2242) -> (fixed-point=w2241:fxp<+,32,32>)  [unwired: 1 in]
        n468 = To Fixed-Point(number=w2213) -> (fixed-point=w2214:fxp<+,32,32>)  [unwired: 1 in]
        n469 = To Fixed-Point(number=w2206) -> (fixed-point=w2205:fxp<+,32,32>)  [unwired: 1 in]
        n470 = To Fixed-Point(number=w2181) -> (fixed-point=w2182:fxp<+,32,32>)  [unwired: 1 in]
        n471 = To Fixed-Point(number=w2174) -> (fixed-point=w2173:fxp<+,32,32>)  [unwired: 1 in]
        n472 = To Fixed-Point(number=w2149) -> (fixed-point=w2150:fxp<+,32,32>)  [unwired: 1 in]
        n473 = feedback #29() -> (w2231:bool)  [unwired: 1 in]
        n474 = And(x=w2230, y=w2231) -> (x .and. y?=w2232:bool)
        n475 = feedback #30() -> (w2224:bool)  [unwired: 1 in]
        n476 = And(x=w2225, y=w2224) -> (x .and. y?=w2223:bool)
        n477 = feedback #31() -> (w2195:bool)  [unwired: 1 in]
        n478 = And(x=w2194, y=w2195) -> (x .and. y?=w2196:bool)
        n479 = feedback #32() -> (w2192:bool)  [unwired: 1 in]
        n480 = And(x=w2193, y=w2192) -> (x .and. y?=w2191:bool)
        n481 = feedback #33() -> (w2163:bool)  [unwired: 1 in]
        n482 = And(x=w2162, y=w2163) -> (x .and. y?=w2164:bool)
        n483 = feedback #34() -> (w2160:bool)  [unwired: 1 in]
        n484 = And(x=w2161, y=w2160) -> (x .and. y?=w2159:bool)
        n485 = xnode "High Throughput Divide"("x"=w2129, "y"=w2241, "input valid"=w2232) -> ("x/y"=w2238:fxp<+,28,17>, "output valid"=w2234:bool, "ready for input"=w2233:bool)  [unwired: 1 in]
        n486 = feedback-in #29(w2233) -> ()
        n487 = xnode "High Throughput Divide"("x"=w2129, "y"=w2214, "input valid"=w2223) -> ("x/y"=w2217:fxp<+,28,17>, "output valid"=w2221:bool, "ready for input"=w2222:bool)  [unwired: 1 in]
        n488 = feedback-in #30(w2222) -> ()
        n489 = xnode "High Throughput Divide"("x"=w2129, "y"=w2205, "input valid"=w2196) -> ("x/y"=w2202:fxp<+,28,17>, "output valid"=w2198:bool, "ready for input"=w2197:bool)  [unwired: 1 in]
        n490 = feedback-in #31(w2197) -> ()
        n491 = xnode "High Throughput Divide"("x"=w2129, "y"=w2182, "input valid"=w2191) -> ("x/y"=w2185:fxp<+,28,17>, "output valid"=w2189:bool, "ready for input"=w2190:bool)  [unwired: 1 in]
        n492 = feedback-in #32(w2190) -> ()
        n493 = xnode "High Throughput Divide"("x"=w2129, "y"=w2173, "input valid"=w2164) -> ("x/y"=w2170:fxp<+,28,17>, "output valid"=w2166:bool, "ready for input"=w2165:bool)  [unwired: 1 in]
        n494 = feedback-in #33(w2165) -> ()
        n495 = xnode "High Throughput Divide"("x"=w2129, "y"=w2150, "input valid"=w2159) -> ("x/y"=w2153:fxp<+,28,17>, "output valid"=w2157:bool, "ready for input"=w2158:bool)  [unwired: 1 in]
        n496 = feedback-in #34(w2158) -> ()
        n497 = Select(t=u32 0 ("f"), s=w2234, f=w2242) -> (s? t:f=w2226:u32)
        n498 = Select(t=u32 0 ("f"), s=w2221, f=w2213) -> (s? t:f=w2142:u32)
        n499 = Select(t=u32 0 ("f"), s=w2198, f=w2206) -> (s? t:f=w2138:u32)
        n500 = Select(t=u32 0 ("f"), s=w2189, f=w2181) -> (s? t:f=w2135:u32)
        n501 = Select(t=u32 0 ("f"), s=w2166, f=w2174) -> (s? t:f=w2130:u32)
        n502 = Select(t=u32 0 ("f"), s=w2157, f=w2149) -> (s? t:f=w2124:u32)
        n503 = To Fixed-Point(fixed-point type=fxp<+/-,28,17> 0.0 ("AI0"), number=w2238) -> (fixed-point=w2236:fxp<+/-,28,17>)
        n504 = To Fixed-Point(fixed-point type=fxp<+/-,28,17> 0.0 ("AI0"), number=w2217) -> (fixed-point=w2219:fxp<+/-,28,17>)
        n505 = To Fixed-Point(fixed-point type=fxp<+/-,28,17> 0.0 ("AI0"), number=w2202) -> (fixed-point=w2200:fxp<+/-,28,17>)
        n506 = To Fixed-Point(fixed-point type=fxp<+/-,28,17> 0.0 ("AI0"), number=w2185) -> (fixed-point=w2187:fxp<+/-,28,17>)
        n507 = To Fixed-Point(fixed-point type=fxp<+/-,28,17> 0.0 ("AI0"), number=w2170) -> (fixed-point=w2168:fxp<+/-,28,17>)
        n508 = To Fixed-Point(fixed-point type=fxp<+/-,28,17> 0.0 ("AI0"), number=w2153) -> (fixed-point=w2155:fxp<+/-,28,17>)
        n509 = Or(x=w2244, y=w2234) -> (x .or. y?=w2239:bool)
        n510 = Or(x=w2211, y=w2221) -> (x .or. y?=w2216:bool)
        n511 = Or(x=w2208, y=w2198) -> (x .or. y?=w2203:bool)
        n512 = Or(x=w2179, y=w2189) -> (x .or. y?=w2184:bool)
        n513 = Or(x=w2176, y=w2166) -> (x .or. y?=w2171:bool)
        n514 = Or(x=w2147, y=w2157) -> (x .or. y?=w2152:bool)
        n515 = Select(t=fxp<+/-,28,17> 0.0 ("AI0"), s=w2244, f=w2236) -> (s? t:f=w2240:fxp<+/-,28,17>)
        n516 = Select(t=fxp<+/-,28,17> 0.0 ("AI0"), s=w2211, f=w2219) -> (s? t:f=w2215:fxp<+/-,28,17>)
        n517 = Select(t=fxp<+/-,28,17> 0.0 ("AI0"), s=w2208, f=w2200) -> (s? t:f=w2204:fxp<+/-,28,17>)
        n518 = Select(t=fxp<+/-,28,17> 0.0 ("AI0"), s=w2179, f=w2187) -> (s? t:f=w2183:fxp<+/-,28,17>)
        n519 = Select(t=fxp<+/-,28,17> 0.0 ("AI0"), s=w2176, f=w2168) -> (s? t:f=w2172:fxp<+/-,28,17>)
        n520 = Select(t=fxp<+/-,28,17> 0.0 ("AI0"), s=w2147, f=w2155) -> (s? t:f=w2151:fxp<+/-,28,17>)
        n521 = Select(t=w2240, s=w2239, f=w2228) -> (s? t:f=w2121:fxp<+/-,28,17>)
        n522 = Select(t=w2215, s=w2216, f=w2143) -> (s? t:f=w2120:fxp<+/-,28,17>)
        n523 = Select(t=w2204, s=w2203, f=w2139) -> (s? t:f=w2119:fxp<+/-,28,17>)
        n524 = Select(t=w2183, s=w2184, f=w2136) -> (s? t:f=w2118:fxp<+/-,28,17>)
        n525 = Select(t=w2172, s=w2171, f=w2131) -> (s? t:f=w2117:fxp<+/-,28,17>)
        n526 = Select(t=w2151, s=w2152, f=w2125) -> (s? t:f=w2116:fxp<+/-,28,17>)
        n527 = Build Array(w2121, w2120, w2119, w2118, w2117, w2116) -> (w2115:fxp<+/-,28,17>[])
      }
    }
    n528 = global write "Diagnostic Global.vi" "Diag_Global"(w1674) -> ()
  }
  n529 = while {
    shift-right: [w2435] -> _
    shift-left: _ -> [w2430]
    stop <- FALSE stop-if-true
    w2422 = refnum<k21> "Signal for Speed"  # FIFO
    # "set at 31.25 kHz"
    n530 = global read "ADC AI Global.vi" "AI16-47"() -> (w2429:fxp<+/-,28,17>[])
    n531 = case shown="1..2500" w2430 {
      tunnel: [fxp<+/-,28,17> -21.0 ("Controller_Current_1 (AI6)") w2475 fxp<+/-,28,17> -22.0 ("Controller_Current_1 (AI6)") w2484 fxp<+/-,28,17> -23.0 ("Controller_Current_1 (AI6)") w2494 fxp<+/-,28,17> -24.0 ("Controller_Current_1 (AI6)") w2503 fxp<+/-,28,17> -25.0 ("Controller_Current_1 (AI6)") w2512 fxp<+/-,28,17> -26.0 ("Controller_Current_1 (AI6)") w2520 fxp<+/-,28,17> -21.5 ("Controller_Current_1 (AI6)") w2529 fxp<+/-,28,17> -22.5 ("Controller_Current_1 (AI6)") w2538 fxp<+/-,28,17> -23.5 ("Controller_Current_1 (AI6)") w2548 fxp<+/-,28,17> -24.5 ("Controller_Current_1 (AI6)") w2557 fxp<+/-,28,17> -25.5 ("Controller_Current_1 (AI6)") w2566 fxp<+/-,28,17> -26.5 ("Controller_Current_1 (AI6)") w2574 fxp<+/-,28,17> -31.0 ("Controller_Current_1 (AI6)")] -> w2426
      tunnel: w2429 -> [_ w2476 _ w2485 _ w2493 _ w2502 _ w2511 _ w2521 _ w2530 _ w2539 _ w2547 _ w2556 _ w2565 _ w2575 _]
      tunnel: [TRUE FALSE TRUE FALSE TRUE FALSE TRUE FALSE TRUE FALSE TRUE FALSE TRUE FALSE TRUE FALSE TRUE FALSE TRUE FALSE TRUE FALSE TRUE FALSE TRUE] -> w2425
      tunnel: "FFT_Amp?" -> [_ w2470 _ w2479 _ w2488 _ w2497 _ w2506 _ w2515 _ w2524 _ w2533 _ w2542 _ w2551 _ w2560 _ w2569 _]
      frame 0, Default {
        # "Start V1"
      }
      frame 1..2500 {
        n532 = Select(t=0 ("index"), s=w2470, f=26) -> (s? t:f=w2472:i32)
        n533 = Index Array(array=w2476, index=w2472) -> (element=w2475:fxp<+/-,28,17>)
      }
      frame 2501 {
        # "Start V2"
      }
      frame 2502..5001 {
        n534 = Select(t=1 ("index"), s=w2479, f=27) -> (s? t:f=w2481:i32)
        n535 = Index Array(array=w2485, index=w2481) -> (element=w2484:fxp<+/-,28,17>)
      }
      frame 5002 {
        # "Start V3"
      }
      frame 5003..7502 {
        n536 = Select(t=2 ("index"), s=w2488, f=28) -> (s? t:f=w2490:i32)
        n537 = Index Array(array=w2493, index=w2490) -> (element=w2494:fxp<+/-,28,17>)
      }
      frame 7503 {
        # "Start V4"
      }
      frame 7504..10003 {
        n538 = Select(t=3 ("index"), s=w2497, f=29) -> (s? t:f=w2499:i32)
        n539 = Index Array(array=w2502, index=w2499) -> (element=w2503:fxp<+/-,28,17>)
      }
      frame 10004 {
        # "Start V5"
      }
      frame 10005..12504 {
        n540 = Select(t=4 ("index"), s=w2506, f=30) -> (s? t:f=w2508:i32)
        n541 = Index Array(array=w2511, index=w2508) -> (element=w2512:fxp<+/-,28,17>)
      }
      frame 12505 {
        # "Start V6"
      }
      frame 12506..15005 {
        n542 = Select(t=5 ("index"), s=w2515, f=31) -> (s? t:f=w2517:i32)
        n543 = Index Array(array=w2521, index=w2517) -> (element=w2520:fxp<+/-,28,17>)
      }
      frame 15006 {
        # "Start V1\nsecond\nread"
      }
      frame 15007..17506 {
        n544 = Select(t=0 ("index"), s=w2524, f=26) -> (s? t:f=w2526:i32)
        n545 = Index Array(array=w2530, index=w2526) -> (element=w2529:fxp<+/-,28,17>)
      }
      frame 17507 {
        # "Start V2\nsecond\nread"
      }
      frame 17508..20007 {
        n546 = Select(t=1 ("index"), s=w2533, f=27) -> (s? t:f=w2535:i32)
        n547 = Index Array(array=w2539, index=w2535) -> (element=w2538:fxp<+/-,28,17>)
      }
      frame 20008 {
        # "Start V3\nSecond\nread"
      }
      frame 20009..22508 {
        n548 = Select(t=2 ("index"), s=w2542, f=28) -> (s? t:f=w2544:i32)
        n549 = Index Array(array=w2547, index=w2544) -> (element=w2548:fxp<+/-,28,17>)
      }
      frame 22509 {
        # "Start V4\nsecond\nread"
      }
      frame 22510..25009 {
        n550 = Select(t=3 ("index"), s=w2551, f=29) -> (s? t:f=w2553:i32)
        n551 = Index Array(array=w2556, index=w2553) -> (element=w2557:fxp<+/-,28,17>)
      }
      frame 25010 {
        # "Start V5\nsecond\nread"
      }
      frame 25011..27510 {
        n552 = Select(t=4 ("index"), s=w2560, f=30) -> (s? t:f=w2562:i32)
        n553 = Index Array(array=w2565, index=w2562) -> (element=w2566:fxp<+/-,28,17>)
      }
      frame 27511 {
        # "Start V6\nsecond\nread"
      }
      frame 27512..30011 {
        n554 = Select(t=5 ("index"), s=w2569, f=31) -> (s? t:f=w2571:i32)
        n555 = Index Array(array=w2575, index=w2571) -> (element=w2574:fxp<+/-,28,17>)
      }
      frame 30012.. {
        # "Hold"
      }
    }
    n556 = xnode "High Throughput Divide"("x"=w2426, "y"=fxp<+,14,14> 13107.0 ("Controller_Current_1 (AI6)")) -> ("x/y"=w2427:fxp<+/-,28,17>)
    n557 = Select(t=w2426, s=w2425, f=w2427) -> (s? t:f=w2424:fxp<+/-,28,17>)
    n558 = To Fixed-Point(fixed-point type=fxp<+/-,25,6> 0.0 ("Controller_Current_1 (AI6)"), number=w2424) -> (fixed-point=w2432:fxp<+/-,25,6>)
    n559 = Increment(x=w2430) -> (x+1=w2436:i32)
    n560 = xnode ("FIFO Write")("Element"=w2432, "Timeout"=0, "FIFO In"=w2422) -> ()  [unwired: 2 out]
    n561 = Greater?(x=w2436, y=31249) -> (0:w2438:bool)
    n562 = call "Wait4"("Count(Ticks)"=u32 1280 ("Count(mSec)")) -> ()  [unwired: 1 out]
    n563 = Select(t=0, s=w2438, f=w2436) -> (s? t:f=w2435:i32)
  }
  n564 = node-c288(w50) -> ()
  n565 = while {
    stop <- FALSE stop-if-true
    n566 = global read "Diagnostic Global.vi" "Diag_Global"() -> (w2579:fxp<+/-,28,17>[])
    n567 = for {
      tunnel: w2579 -> [w2584] mode=indexing
      tunnel: [w2581] -> w2578 mode=indexing
      n568 = Multiply(x=w2584, y=fxp<+/-,28,17> 100.0) -> (x*y=w2582:fxp<+/-,56,34>)
      n569 = To Unsigned Long Integer(number=w2582) -> (unsigned 32bit integer=w2581:u32)
    }
    n570 = global write "Diagnostic Global (U32).vi" "Diag Global (U32)"(w2578) -> ()
  }
  n571 = node-c288(w13) -> ()
  n572 = node-c288(w44) -> ()
